vi "commander2.vi"() -> ()   [LabVIEW 2012]
uses:
  G_SEN.vi
  G_LCM.vi
  G_PATH.vi
  G_VEH.vi
  G_NAV.vi
  G_DATA.vi
  <vilib>/Analysis/Matrix/Datatypes/RealMatrix.ctl
  <vilib>/Analysis/Matrix/NI_Matrix.lvlib
panel:
  in  "gain":dbl=0.7
  out "Waveform Chart 8":dbl(graph)
  out "Waveform Chart 7":dbl(graph)
  out "Waveform Chart 6":dbl(graph)
  in  "save lcm":bool
  out "LCM Recv Data":string
  out "GPS DATA 2":T1={"type"="None", "x_lcc"=-59.06772232055664, "y_lcc"=-26.082616806030273, "latdev"=0.0, "londev"=0.0, "sats"=0, "gps_l1_ranges"=0, "gps_l1_mask_ranges"=0, "gps_l2_mask_ranges"=0, "Heading"=89.78975677490234, "lon"=0.0, "lat"=0.0, "time"="None", "hgps"=89.78975677490234, "lag"=89.78975677490234, "MAP"="None"} {"lag" format="%#_5g"; "hgps" format="%#_5g"; "lat" format="%#_11g"; "lon" format="%#_11g"; "Heading" format="%#_5g"; "latdev" format="%#_4g"; "londev" format="%#_4g"}
  in  "obs":bool
  in  "x":dbl
  in  "log":bool
  out "Waveform Chart 5":dbl(graph)
  in  "y":dbl min=-1.0 max=1.0 step=1.0
  out "x = 0?":bool
  out "timmer 2":u32
  out "timmer":u32
  out "Speed limit":dbl=8.0
  out "collision":bool
  out "Mission":i32=9
  in  "Load WPT":bool
  in  "Max. Vel.":dbl=20.0
  in  "RESET PATH":bool
  out "col":i16(graph)
  out "stop":bool
  in  "Reverse":bool
  in  "STOP":bool
  out "Waveform Chart 4":cluster{"auto":i16, "run":i16}(graph)={"auto"=1, "run"=0}
  out "Waveform Chart 3":T2(graph)={"Steer_input"=10.50986504720403, "Steer_output"=3.6, "handle"=10.50986504720403}
  out "Waveform Chart 2":T3(graph)={"VS_des"=4.606086314285715, "VS_can"=8.738, "VS_des"=5.0237113142857135}
  out "Heading":cluster{"Heading":dbl, "hgps":dbl}(graph)={"Heading"=269.76568785604456, "hgps"=270.2149981902155}
  out "XY Graph 2":cluster{"Y":dbl[], "Y":dbl[]}[](graph)=[{"Y"=[-241.57278442382812], "Y"=[-497.6172790527344]}, {"Y"=array[297 elements], "Y"=array[297 elements]}, {"Y"=array[297 elements], "Y"=array[297 elements]}, {"Y"=[-96.81030887093378], "Y"=[-438.1146154201037]}]
  out "Gauge":cluster{dbl, dbl, dbl}(knob)={4.606086314285715, 8.738, 5.0237113142857135} scale=-20.0..140.0
  out "Meter":cluster{dbl, dbl, dbl}(knob)={10.50986504720403, 3.6, 10.50986504720403} scale=-550.0..550.0
  out "XY Graph":cluster{"Y":dbl[], "Y":dbl[]}[](graph)=[{"Y"=[0.0], "Y"=[1000.0]}, {"Y"=[], "Y"=[]}, {"Y"=[], "Y"=[]}, {"Y"=[55.79381017995934], "Y"=[-143.41137512848826]}, {"Y"=[1.8243630881955273], "Y"=[-0.6091599202647308]}, {"Y"=[60.825233010671326, 56.37330625127248, 55.349089235151354, 59.801015994550255, 60.825233010671326], "Y"=[-144.72018116547483, -142.44414335187238, -144.44751039360185, -146.72354820720435, -144.72018116547483]}, {"Y"=[0.0, 2.210107140854234e-06, 8.840428449730098e-06, 1.9890964154001267e-05, 3.536171391260723e-05, 5.5252677611861145e-05, 7.956385525176302e-05, 0.00010829524660493917, 0.00014144685155770276, 0.0001790186695416196, 0.00022101070067037654, 0.00026742294460291305, 0.00031825540077079495, 0.00037350806894664856, 0.0004331809489031002, 0.0004972740399580289, 0.0005657873416566872, 0.0006387208537717015, 0.0007160745756209508, 0.0007978485066360008, 0.0008840426462484174, 0.0009746569938897665, 0.0010696915488779268, 0.0011691463105307776, 0.0012730212781661976, 0.001381316451102066, 0.0014940318285425747, 0.0016111674095782291, 0.0017327231935269083, 0.0018586991794791174, 0.001989095366525362, 0.00212391175364246, 0.002263148340148291, 0.0024068051247922995, 0.002554882106551304, 0.0027073792846294964, 0.002864296657776322, 0.003025634224741225, 0.003191391984614711, 0.0033615699362599116, 0.003536168078198898, 0.0037151864094084885, 0.003898624928524441, 0.004086483634296201, 0.004278762525359525, 0.004475461600350172, 0.0046765808579039, 0.004882120296656467, 0.0050920799150162566, 0.00530645971150534, 0.005525259684645789, 0.005748479832959674, 0.005976120154741693, 0.006208180648513917, 0.006444661312457356, 0.006685562145094082, 0.006930883144491418, 0.007180624309171435, 0.007434785636974084, 0.007693367126535122, 0.007956368775921874, 0.008223790583087975, 0.008495632546100751, 0.008771894663368585, 0.009052576932504053, 0.00933767935191554, 0.009627201919329309, 0.009921144632812684, 0.010219507490205615, 0.010522290489461739, 0.010829493628421005, 0.011141116904923365, 0.011457160316581394, 0.011777623861462416, 0.012102507536951634, 0.012431811341116372, 0.012765535271228146, 0.013103679325240591, 0.0134462435006526, 0.013793227794963059, 0.014144632205784546, 0.014500456730615952, 0.014860701366956164, 0.015225366112190386, 0.015594450963703821, 0.015967955919109045, 0.0163458809754502, 0.016728226130226176, 0.017114991380822175, 0.017506176724168654, 0.0179017821577645, 0.018301807678767545, 0.018706253284335617, 0.019115118971512857, 0.019528404737457095, 0.01994611057932616, 0.02036823649393682, 0.02079478247856059, 0.021225748530014243, 0.02166113464522823, 0.022100940821246695], "Y"=[0.0, 0.05249999993797367, 0.10499999950378934, 0.15749999832528905, 0.2099999960303148, 0.26249999224670867, 0.31499998660231265, 0.3674999787249688, 0.41999996824251923, 0.472499954782806, 0.5249999379736712, 0.577499917442957, 0.6299998928185055, 0.682499863728159, 0.7349998297997596, 0.7874997906611497, 0.8399997459401715, 0.8924996952646672, 0.9449996382624795, 0.9974995745614504, 1.0499995037894228, 1.1024994255742389, 1.1549993395437415, 1.2074992453257731, 1.2599991425481762, 1.3124990308387938, 1.3649989098254687, 1.4174987791360436, 1.4699986383983614, 1.5224984872402658, 1.574998325289599, 1.6274981521742047, 1.6799979675219257, 1.7324977709606055, 1.784997562118088, 1.837497340622216, 1.8899971061008334, 1.9424968581817836, 1.994996596492911, 2.047496320662059, 2.099996030317072, 2.152495725085793, 2.204995404596067, 2.2574950684757384, 2.309994716352652, 2.3624943478546507, 2.414993962609581, 2.467493560245286, 2.519993140389611, 2.5724927026704023, 2.6249922467155042, 2.6774917721527607, 2.7299912786100196, 2.7824907657151243, 2.834990233095921, 2.887489680380256, 2.939989107195975, 2.9924885131709242, 3.0449878979329497, 3.0974872611098974, 3.1499866023296144, 3.2024859212199472, 3.2549852174087435, 3.3074844905238483, 3.3599837401931105, 3.412482966044377, 3.464982167705495, 3.5174813448043127, 3.5699804969686775, 3.6224796238264374, 3.6749787250054404, 3.7274778001335362, 3.7799768488385714, 3.8324758707483966, 3.884974865490859, 3.9374738326938097, 3.989972771985096, 4.042471682992569, 4.094970565344078, 4.147469418667473, 4.199968242590603, 4.2524670367413195, 4.304965800747474, 4.3574645342369145, 4.409963236837495, 4.4624619081770645, 4.514960547883476, 4.567459155584579, 4.6199577309082285, 4.672456273482274, 4.724954782934569, 4.777453258892966, 4.829951700985317, 4.882450108839476, 4.934948482083297, 4.987446820344632, 5.039945123251335, 5.09244339043126, 5.144941621512262, 5.197439816122197, 5.249937973888915]}, {"Y"=[55.85492946607054, 56.300112183962334, 56.74529490185413, 57.19047761974598, 57.635660337637766, 58.08084305552956, 58.52602577342136, 58.97120849131315, 59.416391209205, 59.8615739270968, 60.306756644988596, 60.75193936288038, 61.197122080772175, 61.64230479866403, 62.087487516555825, 62.532670234447615, 62.97785295233941, 63.423035670231265, 63.86821838812306, 64.31340110601485, 64.75858382390665, 65.20376654179844, 65.64894925969023, 66.09413197758208, 66.53931469547388, 66.98449741336567, 67.42968013125746, 67.87486284914931, 68.3200455670411, 68.7652282849329, 69.2104110028247, 69.65559372071655, 70.10077643860835, 70.54595915650015, 70.99114187439193, 71.43632459228371, 71.88150731017556, 72.32669002806736, 72.77187274595916, 73.21705546385095], "Y"=[-143.26925304077835, -143.49687629901547, -143.72449955725253, -143.95212281548962, -144.17974607372668, -144.40736933196374, -144.63499259020085, -144.8626158484379, -145.090239106675, -145.3178623649121, -145.54548562314918, -145.7731088813862, -146.00073213962332, -146.22835539786038, -146.45597865609744, -146.68360191433456, -146.91122517257162, -147.1388484308087, -147.36647168904577, -147.59409494728285, -147.82171820551994, -148.04934146375703, -148.27696472199406, -148.50458798023115, -148.73221123846827, -148.9598344967053, -149.18745775494241, -149.4150810131795, -149.64270427141656, -149.87032752965362, -150.09795078789074, -150.3255740461278, -150.55319730436486, -150.78082056260195, -151.00844382083903, -151.23606707907612, -151.46369033731318, -151.6913135955503, -151.91893685378736, -152.14656011202442]}, {"Y"=[46.95734422441421, 47.0463827596022, 47.13542129479015, 47.224459829978144, 47.31349836516614, 47.40253690035408, 47.49157543554208, 47.58061397073008, 47.669652505918016, 47.75869104110601, 47.84772957629395, 47.936768111481946, 48.02580664666995, 48.11484518185789, 48.20388371704588, 48.292922252233886, 48.381960787421825, 48.47099932260982, 48.56003785779782, 48.64907639298576, 48.73811492817376, 48.827153463361746, 48.91619199854969, 49.00523053373769, 49.09426906892568, 49.18330760411363, 49.272346139301625, 49.361384674489564, 49.45042320967757, 49.53946174486556, 49.6285002800535, 49.717538815241504, 49.8065773504295, 49.89561588561743, 49.984654420805434, 50.07369295599343, 50.16273149118137, 50.251770026369364, 50.34080856155737, 50.429847096745306, 50.5188856319333, 50.607924167121304, 50.69696270230924, 50.78600123749724, 50.875039772685184, 50.96407830787318, 51.05311684306117, 51.142155378249115, 51.23119391343711, 51.320232448625106, 51.40927098381305, 51.49830951900105, 51.58734805418904, 51.67638658937698, 51.765425124564985, 51.85446365975298, 51.94350219494092, 52.03254073012892, 52.12157926531691, 52.21061780050485, 52.29965633569285, 52.38869487088079, 52.477733406068786, 52.56677194125679, 52.65581047644473, 52.74484901163272, 52.833887546820726, 52.922926082008665, 53.01196461719666, 53.10100315238466, 53.190041687572595, 53.27908022276059, 53.36811875794859, 53.45715729313653, 53.54619582832453, 53.635234363512524, 53.72427289870047, 53.813311433888465, 53.902349969076404, 53.99138850426441, 54.0804270394524, 54.16946557464034, 54.25850410982834, 54.34754264501633, 54.43658118020427, 54.525619715392274, 54.61465825058027, 54.70369678576821, 54.792735320956204, 54.88177385614421, 54.970812391332146, 55.05985092652014, 55.148889461708144, 55.23792799689608, 55.32696653208408, 55.41600506727202, 55.50504360246001, 55.59408213764801, 55.683120672835955, 55.77215920802395, 55.861197743211946, 55.95023627839994, 56.03927481358789, 56.12831334877588, 56.21735188396388, 56.306390419151825, 56.39542895433982, 56.48446748952781, 56.573506024715755, 56.66254455990375, 56.75158309509169, 56.84062163027969, 56.92966016546769, 57.01869870065563, 57.10773723584363, 57.196775771031625, 57.285814306219564, 57.37485284140757, 57.46389137659556, 57.552929911783494, 57.64196844697149, 57.73100698215949, 57.82004551734743, 57.90908405253543, 58.08716112291137, 58.176199658099364, 58.26523819328731, 58.354276728475305, 58.4433152636633, 58.53235379885125, 58.62139233403924, 58.71043086922723, 58.79946940441518, 58.88850793960317, 58.97754647479111, 59.06658500997911, 59.15562354516711, 59.24466208035505, 59.333700615543044, 59.42273915073105, 59.511777685918986, 59.60081622110698, 59.689854756294984, 59.778893291482916, 59.86793182667091, 59.956970361858914, 60.04600889704685, 60.13504743223485, 60.31312450261079, 60.402163037798786, 60.491201572986725, 60.58024010817473, 60.66927864336272, 60.75831717855066, 60.84735571373866, 60.93639424892665, 61.02543278411459, 61.114471319302595, 61.203509854490534, 61.29254838967853, 61.38158692486653, 61.47062546005447, 61.55966399524247, 61.64870253043047, 61.73774106561841, 61.826779600806404, 61.91581813599439, 62.00485667118234, 62.093895206370334, 62.18293374155833, 62.271972276746276, 62.36101081193427, 62.45004934712227, 62.53908788231021, 62.62812641749821, 62.71716495268615, 62.80620348787415, 62.895242023062146, 62.984280558250084, 63.07331909343808, 63.162357628626076, 63.251396163814015, 63.34043469900201, 63.42947323419001, 63.51851176937796, 63.60755030456595, 63.69658883975394, 63.78562737494189, 63.87466591012988, 63.96370444531783, 64.05274298050581, 64.14178151569382, 64.23082005088176, 64.31985858606976, 64.40889712125775, 64.4979356564457, 64.58697419163369, 64.76505126200964, 64.85408979719762, 64.94312833238557, 65.03216686757357, 65.12120540276156, 65.2102439379495, 65.29928247313751, 65.38832100832549, 65.47735954351344, 65.56639807870144, 65.65543661388938, 65.74447514907737, 65.83351368426537, 65.92255221945331, 66.0115907546413, 66.10062928982931, 66.18966782501724, 66.27870636020525, 66.36774489539324, 66.45678343058118, 66.54582196576918, 66.63486050095719, 66.72389903614511, 66.81293757133312, 66.9019761065211, 66.99101464170904, 67.08005317689705, 67.16909171208498, 67.25813024727299, 67.34716878246098, 67.43620731764892, 67.52524585283692, 67.61428438802493, 67.70332292321285, 67.79236145840086, 67.88139999358886, 67.97043852877678, 68.05947706396479, 68.14851559915279, 68.23755413434073, 68.32659266952872, 68.41563120471668, 68.50466973990466, 68.59370827509267, 68.6827468102806, 68.7717853454686, 68.8608238806566, 68.94986241584455, 69.03890095103253, 69.12793948622053, 69.21697802140848, 69.30601655659646, 69.39505509178447, 69.48409362697241, 69.5731321621604, 69.6621706973484, 69.75120923253635, 69.84024776772434, 69.92928630291229, 70.01832483810027, 70.10736337328828, 70.19640190847622, 70.2854404436642, 70.37447897885221, 70.46351751404015, 70.55255604922814, 70.64159458441614, 70.7306331196041, 70.81967165479207, 70.90871018998008, 70.99774872516802, 71.08678726035602, 71.17582579554401, 71.26486433073195, 71.35390286591995, 71.44294140110789, 71.5319799362959, 71.62101847148388, 71.71005700667183, 71.79909554185983, 71.88813407704782, 71.97717261223576, 72.06621114742377, 72.15524968261175, 72.2442882177997, 72.3333267529877, 72.42236528817568, 72.51140382336364, 72.60044235855163, 72.68948089373963, 72.77851942892757, 72.86755796411556, 72.9565964993035, 73.04563503449151, 73.13467356967949, 73.22371210486745, 73.31275064005544, 73.40178917524342, 73.49082771043138, 73.57986624561937], "Y"=[-138.89375124553214, -138.93927200180423, -138.98479275807625, -139.0303135143483, -139.07583427062036, -139.12135502689242, -139.16687578316444, -139.21239653943653, -139.25791729570855, -139.30343805198058, -139.34895880825266, -139.3944795645247, -139.44000032079677, -139.4855210770688, -139.53104183334085, -139.5765625896129, -139.62208334588496, -139.667604102157, -139.71312485842907, -139.7586456147011, -139.80416637097318, -139.8496871272452, -139.89520788351723, -139.9407286397893, -139.98624939606134, -140.0317701523334, -140.07729090860545, -140.1228116648775, -140.16833242114956, -140.2138531774216, -140.25937393369364, -140.30489468996572, -140.35041544623775, -140.39593620250977, -140.44145695878186, -140.48697771505388, -140.53249847132597, -140.578019227598, -140.62353998387005, -140.66906074014207, -140.71458149641416, -140.76010225268618, -140.80562300895826, -140.8511437652303, -140.89666452150234, -140.9421852777744, -140.98770603404643, -141.0332267903185, -141.07874754659053, -141.1242683028626, -141.16978905913462, -141.2153098154067, -141.26083057167872, -141.3063513279508, -141.35187208422283, -141.3973928404949, -141.44291359676694, -141.48843435303897, -141.53395510931105, -141.57947586558308, -141.62499662185516, -141.67051737812716, -141.71603813439924, -141.76155889067127, -141.80707964694335, -141.85260040321535, -141.89812115948743, -141.94364191575949, -141.9891626720315, -142.0346834283036, -142.08020418457562, -142.1257249408477, -142.1712456971197, -142.21676645339178, -142.2622872096638, -142.3078079659359, -142.3533287222079, -142.39884947847997, -142.44437023475203, -142.48989099102408, -142.53541174729614, -142.58093250356816, -142.62645325984025, -142.67197401611224, -142.71749477238433, -142.76301552865635, -142.80853628492844, -142.85405704120046, -142.89957779747255, -142.94509855374454, -142.99061931001663, -143.03614006628868, -143.0816608225607, -143.1271815788328, -143.17270233510482, -143.2182230913769, -143.2637438476489, -143.30926460392098, -143.354785360193, -143.4003061164651, -143.4458268727371, -143.4913476290092, -143.5368683852812, -143.58238914155328, -143.62790989782533, -143.67343065409736, -143.71895141036944, -143.76447216664147, -143.80999292291352, -143.85551367918555, -143.90103443545763, -143.94655519172966, -143.99207594800174, -144.03759670427374, -144.08311746054582, -144.12863821681785, -144.1741589730899, -144.21967972936199, -144.265200485634, -144.3107212419061, -144.3562419981781, -144.40176275445017, -144.4472835107222, -144.49280426699428, -144.58384577953836, -144.6293665358104, -144.67488729208247, -144.72040804835453, -144.76592880462653, -144.81144956089864, -144.85697031717064, -144.90249107344272, -144.94801182971474, -144.99353258598683, -145.03905334225882, -145.0845740985309, -145.13009485480293, -145.17561561107502, -145.22113636734704, -145.2666571236191, -145.31217787989118, -145.35769863616318, -145.40321939243526, -145.4487401487073, -145.49426090497937, -145.5397816612514, -145.58530241752348, -145.63082317379548, -145.7218646863396, -145.76738544261164, -145.8129061988837, -145.85842695515572, -145.90394771142783, -145.94946846769983, -145.9949892239719, -146.04050998024394, -146.08603073651602, -146.13155149278802, -146.1770722490601, -146.22259300533213, -146.2681137616042, -146.31363451787624, -146.3591552741483, -146.40467603042035, -146.45019678669237, -146.49571754296446, -146.54123829923648, -146.58675905550857, -146.6322798117806, -146.67780056805265, -146.72332132432467, -146.76884208059676, -146.81436283686878, -146.85988359314084, -146.9054043494129, -146.95092510568492, -146.99644586195703, -147.04196661822903, -147.0874873745011, -147.13300813077313, -147.17852888704522, -147.22404964331722, -147.2695703995893, -147.31509115586132, -147.3606119121334, -147.40613266840543, -147.4516534246775, -147.49717418094954, -147.54269493722157, -147.58821569349365, -147.63373644976568, -147.67925720603776, -147.72477796230976, -147.77029871858184, -147.81581947485387, -147.86134023112595, -147.90686098739798, -147.9979024999421, -148.0434232562141, -148.08894401248617, -148.13446476875822, -148.17998552503028, -148.22550628130233, -148.27102703757438, -148.3165477938464, -148.3620685501185, -148.40758930639052, -148.45311006266255, -148.49863081893463, -148.54415157520666, -148.58967233147874, -148.63519308775076, -148.6807138440228, -148.72623460029487, -148.77175535656693, -148.81727611283895, -148.86279686911104, -148.90831762538306, -148.95383838165512, -148.99935913792717, -149.0448798941992, -149.09040065047128, -149.1359214067433, -149.18144216301536, -149.22696291928742, -149.27248367555944, -149.31800443183153, -149.36352518810358, -149.4090459443756, -149.4545667006477, -149.50008745691972, -149.54560821319174, -149.59112896946382, -149.63664972573585, -149.68217048200793, -149.72769123827996, -149.77321199455199, -149.81873275082407, -149.86425350709612, -149.90977426336815, -149.95529501964023, -150.00081577591226, -150.0463365321843, -150.09185728845637, -150.1373780447284, -150.18289880100048, -150.2284195572725, -150.27394031354456, -150.3194610698166, -150.36498182608864, -150.4105025823607, -150.45602333863278, -150.5015440949048, -150.54706485117688, -150.5925856074489, -150.63810636372094, -150.68362711999302, -150.72914787626505, -150.7746686325371, -150.82018938880915, -150.86571014508118, -150.91123090135326, -150.9567516576253, -151.00227241389734, -151.04779317016943, -151.09331392644145, -151.13883468271348, -151.18435543898556, -151.2298761952576, -151.27539695152967, -151.3209177078017, -151.36643846407375, -151.4119592203458, -151.45747997661783, -151.5030007328899, -151.54852148916194, -151.594042245434, -151.63956300170608, -151.6850837579781, -151.73060451425013, -151.77612527052221, -151.82164602679424, -151.8671667830663, -151.91268753933835, -151.95820829561038, -152.00372905188246, -152.04924980815449, -152.09477056442654, -152.14029132069862, -152.18581207697065, -152.23133283324267, -152.27685358951476, -152.32237434578678, -152.36789510205887, -152.4134158583309, -152.45893661460295, -152.504457370875]}, {"Y"=[], "Y"=[]}, {"Y"=[], "Y"=[]}, {"Y"=[], "Y"=[]}, {"Y"=[-16.5, -15.25, -15.0, -13.5, -13.25, -13.25, -13.25, -13.0, -13.0, -12.75, -12.75, -12.75, -12.75, -12.75, -12.75, -12.75, -12.5, -12.5, -12.5, -12.5, -12.5, -12.5, -12.25, -12.25, -12.25, -12.25, -12.25, -12.25, -12.0, -12.0, -12.0, -11.75, -11.75, -11.75, -11.5, -11.5, -11.5, -11.5, -11.5, -11.25, -10.75, -10.75, -10.5, -10.5, -10.25, -10.25, -10.0, -10.0, -10.0, -10.0, -10.0, -9.75, -9.75, -9.75, -9.75, -9.75, -9.75, -9.75, -9.75, -9.75, -9.75, -9.5, -9.5, -9.5, -9.5, -9.5, -9.5, -9.5, -9.5, -9.5, -9.5, -9.5, -9.5, -9.5, -9.5, -9.5, -9.5, -9.5, -9.5, -9.5, -9.25, -9.25, -9.25, -9.25, -9.25, -9.25, -9.25, -9.25, -9.25, -9.25, -9.25, -9.25, -9.25, -9.25, -9.25, -9.25, -9.25, -9.25, -9.25, -9.25, -9.25, -9.25, -9.0, -9.0, -9.0, -9.0, -9.0, -9.0, -9.0, -9.0, -9.0, -9.0, -9.0, -9.0, -9.0, -9.0, -9.0, -9.0, -9.0, -9.0, -9.0, -9.0, -9.0, -9.0, -9.0, -9.0, -9.0, -9.0, -8.75, -8.75, -8.75, -8.75, -8.75, -8.75, -8.75, -8.75, -8.75, -8.75, -8.75, -8.75, -8.75, -8.75, -8.75, -8.75, -8.75, -8.75, -8.75, -8.75, -8.75, -8.75, -8.75, -8.75, -8.75, -8.75, -8.75, -8.75, -8.75, -8.75, -8.75, -8.75, -8.75, -8.75, -8.75, -8.75, -8.75, -8.5, -8.5, -8.5, -8.5, -8.5, -8.5, -8.5, -8.5, -8.5, -8.5, -8.5, -8.5, -8.5, -8.5, -8.5, -8.5, -8.5, -8.5, -8.5, -8.5, -8.5, -8.5, -8.5, -8.5, -8.5, -8.5, -8.5, -8.5, -8.5, -8.5, -8.5, -8.5, -8.5, -8.5, -8.5, -8.5, -8.25, -8.25, -8.25, -8.25, -8.25, -8.25, -8.25, -8.25, -8.25, -8.25, -8.25, -8.25, -8.25, -8.25, -8.25, -8.25, -8.25, -8.25, -8.25, -8.25, -8.25, -8.25, -8.25, -8.25, -8.25, -8.25, -8.25, -8.25, -8.25, -8.25, -8.25, -8.25, -8.25, -8.0, -8.0, -8.0, -8.0, -8.0, -8.0, -8.0, -8.0, -8.0, -8.0, -8.0, -8.0, -8.0, -8.0, -8.0, -8.0, -8.0, -8.0, -8.0, -8.0, -8.0, -8.0, -8.0, -8.0, -8.0, -7.75, -7.75, -7.75, -7.75, -7.75, -7.75, -7.75, -7.75, -7.75, -7.75, -7.75, -7.75, -7.75, -7.75, -7.75, -7.75, -7.75, -7.75, -7.75, -7.75, -7.75, -7.75, -7.75, -7.75, -7.75, -7.75, -7.5, -7.5, -7.5, -7.5, -7.5, -7.5, -7.5, -7.5, -7.5, -7.5, -7.5, -7.5, -7.5, -7.5, -7.5, -7.5, -7.5, -7.5, -7.5, -7.5, -7.5, -7.5, -7.5, -7.5, -7.5, -7.25, -7.25, -7.25, -7.25, -7.25, -7.25, -7.25, -7.25, -7.25, -7.25, -7.25, -7.25, -7.25, -7.25, -7.25, -7.25, -7.25, -7.25, -7.25, -7.25, -7.25, -7.25, -7.25, -7.0, -7.0, -7.0, -7.0, -7.0, -7.0, -7.0, -7.0, -7.0, -7.0, -7.0, -7.0, -7.0, -7.0, -7.0, -7.0, -7.0, -7.0, -7.0, -6.75, -6.75, -6.75, -6.75, -6.75, -6.75, -6.75, -6.75, -6.75, -6.75, -6.75, -6.75, -6.75, -6.75, -6.75, -6.75, -6.75, -6.75, -6.75, -6.75, -6.75, -6.75, -6.75, -6.5, -6.5, -6.5, -6.5, -6.5, -6.5, -6.5, -6.5, -6.5, -6.5, -6.5, -6.5, -6.5, -6.5, -6.5, -6.5, -6.5, -6.5, -6.5, -6.5, -6.5, -6.5, -6.5, -6.5, -6.5, -6.5, -6.5, -6.5, -6.5, -6.5, -6.25, -6.25, -6.25, -6.25, -6.25, -6.25, -6.25, -6.25, -6.25, -6.25, -6.25, -6.25, -6.25, -6.25, -6.25, -6.25, -6.25, -6.0, -6.0, -6.0, -6.0, -6.0, -6.0, -6.0, -6.0, -6.0, -6.0, -6.0, -5.75, -5.75, -5.75, -5.75, -5.75, -5.75, -5.75, -5.75, -5.75, -5.75, -5.5, -5.25, -5.0, -4.75, -4.5, -4.5, -4.25, -4.25, -4.0, -4.0, -3.75, -3.75, -3.5, -3.5, -3.25, -3.25, -3.25, -3.25, -3.0, -3.0, 2.0, 2.0, 2.0, 2.0, 2.0, 2.0, 2.0, 2.25, 2.25, 2.25, 2.25, 2.25, 2.25, 2.25, 2.25, 2.25, 2.25, 2.25, 2.25, 2.25, 2.25, 2.25, 2.25, 2.25, 2.25, 2.25, 2.25, 2.25, 2.25, 2.5, 2.5, 2.5, 2.5, 2.5, 2.5, 2.5, 2.5, 2.5, 2.5, 2.5, 2.5, 2.5, 2.5, 2.5, 2.5, 2.5, 2.5, 2.5, 2.5, 2.5, 2.5, 2.5, 2.5, 2.5, 2.5, 2.5, 2.5, 2.5, 2.5, 2.5, 2.5, 2.5, 2.5, 2.5, 2.5, 2.5, 2.5, 2.5, 2.5, 2.5, 2.5, 2.75, 2.75, 2.75, 2.75, 2.75, 2.75, 2.75, 2.75, 2.75, 2.75, 2.75, 2.75, 2.75, 2.75, 2.75, 2.75, 2.75, 2.75, 2.75, 2.75, 2.75, 2.75, 2.75, 2.75, 2.75, 2.75, 2.75, 2.75, 2.75, 2.75, 2.75, 2.75, 2.75, 2.75, 2.75, 2.75, 2.75, 2.75, 2.75, 2.75, 2.75, 2.75, 2.75, 2.75, 2.75, 2.75, 2.75, 2.75, 2.75, 2.75, 3.0, 3.0, 3.0, 3.0, 3.0, 3.0, 3.0, 3.0, 3.0, 3.0, 3.0, 3.0, 3.0, 3.0, 3.0, 3.0, 3.0, 3.0, 3.0, 3.0, 3.0, 3.0, 3.0, 3.0, 3.0, 3.0, 3.0, 3.0, 3.0, 3.0, 3.0, 3.0, 3.0, 3.0, 3.0, 3.0, 3.0, 3.0, 3.0, 3.0, 3.0, 3.0, 3.0, 3.0, 3.0, 3.0, 3.0, 3.25, 3.25, 3.25, 3.25, 3.25, 3.25, 3.25, 3.25, 3.25, 3.25, 3.25, 3.25, 3.25, 3.25, 3.25, 3.25, 3.25, 3.25, 3.25, 3.25, 3.25, 3.25, 3.25, 3.25, 3.25, 3.25, 3.25, 3.25, 3.25, 3.25, 3.25, 3.25, 3.25, 3.25, 3.25, 3.25, 3.25, 3.25, 3.25, 3.25, 3.25, 3.25, 3.25, 3.25, 3.25, 3.25, 3.25, 3.25, 3.25, 3.25, 3.25, 3.25, 3.25, 3.5, 3.5, 3.5, 3.5, 3.5, 3.5, 3.5, 3.5, 3.5, 3.5, 3.5, 3.5, 3.5, 3.5, 3.5, 3.5, 3.5, 3.5, 3.5, 3.5, 3.5, 3.5, 3.5, 3.5, 3.5, 3.5, 3.5, 3.5, 3.5, 3.5, 3.5, 3.5, 3.5, 3.5, 3.5, 3.5, 3.5, 3.5, 3.5, 3.5, 3.5, 3.5, 3.5, 3.5, 3.5, 3.5, 3.5, 3.5, 3.5, 3.5, 3.5, 3.5, 3.5, 3.5, 3.5, 3.5, 3.5, 3.75, 3.75, 3.75, 3.75, 3.75, 3.75, 3.75, 3.75, 3.75, 3.75, 3.75, 3.75, 3.75, 3.75, 3.75, 3.75, 3.75, 3.75, 3.75, 3.75, 3.75, 3.75, 3.75, 3.75, 3.75, 3.75, 3.75, 3.75, 3.75, 3.75, 3.75, 3.75, 3.75, 3.75, 3.75, 3.75, 3.75, 4.0, 4.0, 4.0, 4.0, 4.0, 4.0, 4.0, 4.0, 4.0, 4.0, 4.0, 4.0, 4.0, 4.0, 4.0, 4.0, 4.0, 4.0, 4.0, 4.0, 4.0, 4.0, 4.0, 4.0, 4.0, 4.0, 4.0, 4.0, 4.0, 4.0, 4.0, 4.0, 4.0, 4.0, 4.0, 4.0, 4.25, 4.25, 4.25, 4.25, 4.25, 4.25, 4.25, 4.25, 4.25, 4.25, 4.25, 4.25, 4.25, 4.25, 4.25, 4.25, 4.25, 4.25, 4.25, 4.25, 4.25, 4.25, 4.25, 4.25, 4.25, 4.25, 4.25, 4.25, 4.25, 4.25, 4.25, 4.25, 4.25, 4.25, 4.25, 4.25, 4.25, 4.25, 4.25, 4.25, 4.25, 4.25, 4.25, 4.5, 4.5, 4.5, 4.5, 4.5, 4.5, 4.5, 4.5, 4.5, 4.5, 4.5, 4.5, 4.5, 4.5, 4.5, 4.5, 4.5, 4.5, 4.5, 4.5, 4.5, 4.5, 4.5, 4.5, 4.5, 4.5, 4.5, 4.75, 4.75, 4.75, 4.75, 4.75, 4.75, 4.75, 4.75, 4.75, 4.75, 4.75, 4.75, 4.75, 4.75, 4.75, 4.75, 4.75, 4.75, 4.75, 4.75, 4.75, 4.75, 4.75, 4.75, 4.75, 4.75, 4.75, 4.75, 4.75, 5.0, 5.0, 5.0, 5.0, 5.0, 5.0, 5.0, 5.0, 5.0, 5.0, 5.0, 5.0, 5.0, 5.0, 5.0, 5.0, 5.0, 5.0, 5.0, 5.0, 5.0, 5.25, 5.25, 5.25, 5.25, 5.25, 5.25, 5.25, 5.25, 5.25, 5.25, 5.25, 5.25, 5.25, 5.25, 5.5, 5.5, 5.5, 5.5, 5.5, 5.5, 5.5, 5.5, 5.5, 5.5, 5.5, 5.5, 5.75, 5.75, 5.75, 5.75, 5.75, 5.75, 5.75, 5.75, 5.75, 5.75, 5.75, 5.75, 5.75, 5.75, 5.75, 5.75, 5.75, 6.0, 6.0, 6.0, 6.0, 6.0, 6.0, 6.0, 6.0, 6.0, 6.0, 6.0, 6.25, 6.25, 6.25, 6.25, 6.25, 6.25, 6.25, 6.25, 6.5, 6.5, 6.5, 6.5, 6.5, 6.5, 6.5, 6.5, 6.5, 6.75, 6.75, 6.75, 6.75, 7.0, 7.0, 7.0, 7.25, 7.25, 7.25, 7.25, 7.25, 7.25, 7.25, 7.5, 7.5, 8.0, 8.0, 8.0, 8.0, 8.0, 8.25, 8.25, 8.5, 8.5, 8.5, 8.75, 8.75, 8.75, 8.75, 8.75, 9.0, 9.0, 9.0, 9.0, 9.0, 9.0, 9.25, 9.25, 9.25, 9.25, 9.25, 9.25, 9.5, 9.5, 9.5, 9.5, 9.5, 9.5, 9.75, 9.75, 9.75, 10.0, 10.0, 10.0, 10.0, 10.25, 10.25, 10.5, 10.5, 10.5, 10.75, 10.75, 10.75, 10.75, 11.0, 11.0, 11.0, 11.0, 11.0, 11.25, 11.25, 11.25, 11.25, 11.25, 11.25, 11.25, 11.25, 11.25, 11.25, 11.5, 11.5, 11.5, 11.5, 11.5, 11.5, 11.5, 11.5, 11.5, 11.5, 11.5, 11.5, 11.5, 11.5, 11.5, 11.75, 11.75, 11.75, 11.75, 11.75, 11.75, 11.75, 11.75, 11.75, 11.75, 11.75, 11.75, 11.75, 11.75, 11.75, 11.75, 11.75, 11.75, 11.75, 11.75, 12.0, 12.0, 12.0, 12.0, 12.0, 12.0, 12.0, 12.0, 12.0, 12.0, 12.0, 12.0, 12.0, 12.0, 12.0, 12.0, 12.0, 12.0, 12.0, 12.0, 12.0, 12.0, 12.0, 12.0, 12.0, 12.0, 12.0, 12.25, 12.25, 12.25, 12.25, 12.25, 12.25, 12.25, 12.25, 12.25, 12.25, 12.25, 12.25, 12.25, 12.25, 12.25, 12.25, 12.5, 12.5, 12.5, 12.5, 12.5, 12.5, 12.5, 12.5, 12.5, 12.5, 12.5, 12.5, 12.5, 12.75, 12.75, 12.75, 12.75, 12.75, 12.75, 12.75, 12.75, 12.75, 12.75, 13.0, 13.0, 13.0, 13.0, 13.0, 13.0, 13.0, 13.0, 13.0, 13.0, 13.0, 13.0, 13.0, 13.0, 13.0, 13.0, 13.0, 13.0, 13.0, 13.0, 13.0, 13.0, 13.0, 13.25, 13.25, 13.25, 13.25, 13.25, 13.25, 13.25, 13.25, 13.25, 13.25, 13.25, 13.25, 13.25, 13.25, 13.25, 13.25, 13.25, 13.25, 13.25, 13.5, 13.5, 13.5, 13.5, 13.5, 13.5, 13.5, 13.5, 13.5, 13.5, 13.75, 13.75, 13.75, 13.75, 13.75, 13.75, 13.75, 13.75, 13.75, 14.0, 14.0, 14.0, 14.0, 14.5, 14.75, 15.5, 15.75, 16.0, 19.25, 19.25, 19.25, 19.5, 19.5, 19.75, 22.25, 22.25, 22.25, 22.5, 22.5, 22.5, 22.75, 22.75, 22.75, 22.75, 23.0, 23.0, 23.0, 23.25, 23.25, 23.25, 23.5, 23.5, 23.5, 23.5, 23.5, 23.5, 23.75, 23.75, 23.75, 23.75, 23.75, 23.75, 23.75, 23.75, 23.75, 23.75, 23.75, 24.0, 24.0, 24.0, 24.0, 24.0, 24.0, 24.0, 24.25, 24.25, 24.5], "Y"=[46.5, 46.5, 46.5, 2.75, 0.5, 2.75, 17.0, 0.75, 17.25, -6.5, -2.25, -1.75, 0.5, 0.75, 1.0, 3.75, -6.5, 0.75, 4.0, 4.25, 17.25, 21.5, -6.75, -6.5, -1.75, 17.25, 21.5, 22.25, -6.75, 21.75, 22.0, -6.5, 11.25, 22.0, 10.5, 10.75, 11.0, 11.5, 11.75, -6.0, 3.75, 8.25, -1.0, 8.25, -1.25, -1.0, -7.0, -1.25, 2.75, 3.0, 3.5, -10.75, -10.5, -10.0, -9.5, -9.25, -8.25, -6.75, -1.25, 3.0, 3.25, -20.5, -15.5, -15.25, -14.75, -10.5, -10.25, -10.0, -9.75, -9.25, -9.0, -8.75, -8.25, -8.0, -7.75, -7.5, -1.0, 0.5, 1.5, 2.75, -20.25, -18.25, -17.75, -17.5, -17.0, -15.75, -15.5, -10.75, -10.25, -9.5, -9.0, -8.75, -8.25, -8.0, -7.75, 0.75, 1.0, 1.25, 2.25, 3.5, 7.25, 7.5, -19.0, -17.5, -17.25, -10.5, -10.25, -10.0, -9.25, -9.0, -8.75, -8.25, -8.0, -7.25, -7.0, -6.75, -4.75, -4.5, -4.25, 0.75, 1.0, 1.25, 1.75, 2.25, 2.5, 2.75, 3.5, 7.5, -17.5, -12.75, -12.0, -11.75, -10.5, -9.75, -9.5, -9.25, -9.0, -8.75, -8.5, -8.25, -8.0, -7.75, -7.5, -7.0, -6.75, -4.75, -4.5, -3.75, -3.25, -3.0, -1.5, -0.5, -0.25, 0.0, 0.25, 1.75, 2.5, 2.75, 4.25, 4.75, 5.5, 5.75, 6.25, 7.5, 7.75, -13.25, -13.0, -12.75, -12.0, -11.75, -8.25, -8.0, -7.0, -6.75, -5.5, -5.0, -4.75, -4.5, -4.0, -3.75, -3.25, -3.0, -2.75, -2.0, -1.75, -1.5, -1.0, -0.5, -0.25, 0.0, 0.25, 0.5, 0.75, 1.75, 2.0, 4.0, 4.25, 4.75, 5.75, 6.0, 6.25, -17.5, -12.75, -12.0, -11.5, -10.25, -8.25, -8.0, -7.75, -5.5, -4.75, -4.0, -3.75, -3.5, -3.25, -3.0, -2.75, -2.5, -2.25, -2.0, -1.75, -1.5, -0.75, -0.5, -0.25, 0.0, 0.25, 0.5, 2.25, 4.5, 4.75, 5.75, 6.0, 6.25, -13.5, -13.25, -13.0, -7.75, -5.75, -5.5, -5.25, -5.0, -4.75, -4.5, -3.75, -3.5, -3.25, -2.25, -2.0, -1.75, -1.5, -1.25, -0.75, -0.5, -0.25, 0.0, 0.25, 0.5, 0.75, -13.25, -12.5, -6.0, -5.75, -5.25, -5.0, -4.75, -4.5, -4.25, -3.25, -2.5, -2.25, -2.0, -1.75, -1.5, -1.25, -0.75, -0.5, -0.25, 0.0, 0.25, 0.5, 4.0, 4.25, 7.75, 8.0, -14.0, -13.25, -13.0, -8.0, -5.25, -5.0, -4.75, -3.75, -3.0, -2.0, -1.75, -1.5, -1.25, -0.5, -0.25, 0.25, 0.5, 0.75, 1.0, 1.25, 1.5, 2.25, 2.5, 3.75, 9.25, -7.75, -7.25, -7.0, -6.75, -6.5, -6.25, -6.0, -5.75, -5.5, -5.25, -5.0, -3.5, -1.75, -1.5, -1.25, -0.5, -0.25, 1.0, 1.25, 1.75, 2.5, 5.75, 8.5, -9.0, -8.0, -7.75, -7.0, -6.75, -6.5, -5.5, -5.25, -5.0, -2.0, -1.75, 1.25, 1.5, 2.5, 4.0, 4.25, 4.5, 6.0, 8.5, -9.25, -9.0, -7.5, -7.25, -5.75, -5.5, -2.75, -2.5, -1.0, -0.75, -0.5, -0.25, 0.0, 1.0, 1.25, 1.75, 2.75, 3.0, 4.5, 4.75, 5.75, 6.0, 6.25, -20.0, -8.0, -7.5, -7.25, -4.5, -4.25, -3.25, -3.0, -2.75, -2.5, -1.25, -1.0, -0.75, -0.5, 2.25, 2.5, 2.75, 3.0, 3.25, 3.5, 3.75, 4.0, 4.25, 4.5, 4.75, 5.0, 5.25, 5.5, 5.75, 6.0, -20.25, -20.0, -14.0, -13.75, -8.0, -7.75, -7.25, -5.0, -4.75, -4.5, -3.5, -3.25, -3.0, -2.0, -1.75, -1.5, 3.0, -20.0, -14.0, -13.75, -8.0, -7.75, -7.5, -7.25, -5.0, -2.0, -1.75, -1.5, -20.5, -20.25, -14.25, -8.0, -7.75, -7.5, -2.0, -1.75, -1.5, 3.0, 3.0, 3.0, 3.0, 3.0, 3.0, 20.75, 3.0, 20.75, 3.0, 20.75, 3.0, 20.75, 3.0, 20.75, 3.0, 21.0, 22.0, 22.25, 3.0, 22.25, -8.25, -8.0, -7.25, -2.75, -2.5, -2.25, -2.0, -20.5, -14.5, -14.25, -8.5, -8.25, -8.0, -7.75, -7.25, -4.5, -4.0, -3.5, -3.25, -3.0, -2.5, -2.25, -2.0, -1.5, -1.25, -1.0, 4.75, 6.0, 6.25, -20.5, -20.25, -14.25, -8.25, -8.0, -7.75, -5.0, -4.5, -4.25, -4.0, -3.75, -3.5, -3.25, -3.0, -2.75, -2.5, -2.25, -2.0, -1.75, -1.5, -1.25, -1.0, -0.75, 0.75, 1.75, 2.0, 2.25, 2.5, 2.75, 3.0, 3.25, 3.5, 3.75, 4.0, 5.0, 5.25, 5.5, 5.75, 6.25, 6.5, 6.75, 7.0, -20.5, -20.25, -14.25, -8.25, -7.75, -4.75, -4.5, -4.25, -4.0, -3.75, -3.5, -3.25, -3.0, -2.75, -2.5, -2.0, -1.75, -1.5, -1.25, -1.0, -0.75, -0.5, 0.25, 0.5, 0.75, 1.0, 1.25, 1.5, 1.75, 2.0, 2.25, 2.5, 2.75, 3.25, 3.5, 3.75, 4.0, 4.25, 4.5, 4.75, 5.0, 5.25, 5.5, 5.75, 6.0, 6.25, 6.5, 6.75, 7.0, 7.25, -20.25, -7.75, -5.25, -4.5, -4.25, -4.0, -3.75, -3.5, -3.25, -2.75, -2.5, -2.25, -2.0, -1.75, -1.5, -1.25, -1.0, -0.75, -0.5, -0.25, 0.0, 0.25, 0.5, 0.75, 1.0, 1.25, 1.5, 1.75, 2.0, 2.25, 2.5, 2.75, 4.25, 4.5, 4.75, 5.0, 5.25, 5.5, 5.75, 6.0, 6.25, 6.5, 6.75, 7.0, 7.5, 9.5, 10.75, -20.5, -7.5, -6.75, -6.0, -5.75, -5.0, -4.75, -4.5, -4.25, -4.0, -3.25, -3.0, -2.75, -2.5, -2.0, -1.75, -1.5, -1.25, -1.0, -0.75, -0.5, -0.25, 0.0, 0.25, 0.5, 0.75, 1.0, 1.25, 1.5, 1.75, 2.0, 2.25, 2.5, 2.75, 3.0, 4.5, 4.75, 5.0, 5.25, 5.5, 5.75, 6.0, 6.25, 6.5, 6.75, 7.0, 7.25, 9.25, 9.5, 10.75, 11.0, 12.25, 12.75, -7.75, -7.5, -6.75, -6.5, -5.75, -5.5, -5.25, -4.75, -4.25, -4.0, -3.5, -3.0, -2.75, -2.25, -2.0, -1.75, -1.5, -1.25, -1.0, -0.75, -0.5, -0.25, 0.0, 0.25, 0.5, 0.75, 1.0, 1.25, 1.5, 1.75, 2.0, 2.25, 2.5, 2.75, 3.0, 4.75, 5.0, 5.25, 5.5, 5.75, 6.0, 6.5, 6.75, 7.0, 8.75, 9.0, 9.25, 10.25, 10.75, 11.0, 11.25, 12.25, 12.5, 12.75, 13.0, 13.25, 13.75, -8.75, -7.5, -6.5, -6.25, -5.5, -5.0, -4.75, -4.5, -4.25, -4.0, -2.25, -1.75, -1.5, -1.25, -1.0, -0.75, -0.5, -0.25, 0.0, 0.25, 0.5, 1.0, 1.25, 1.5, 1.75, 2.0, 2.25, 2.5, 2.75, 3.0, 3.25, 9.75, 11.0, 11.25, 12.25, 12.5, 13.0, -8.5, -7.5, -6.75, -6.5, -5.5, -5.25, -4.25, -4.0, -3.25, -3.0, -2.75, -2.5, -2.25, -1.75, -1.5, -1.25, -1.0, -0.75, -0.5, -0.25, 0.0, 0.25, 0.5, 0.75, 1.0, 1.25, 1.5, 1.75, 2.0, 2.25, 2.5, 2.75, 3.0, 12.5, 13.0, 13.25, -9.75, -9.5, -9.25, -8.75, -8.5, -8.25, -7.75, -7.5, -7.25, -7.0, -6.75, -6.5, -6.25, -6.0, -5.75, -5.0, -4.25, -3.0, -2.75, -2.5, -2.25, -1.75, -1.5, 0.0, 0.25, 0.5, 0.75, 1.0, 1.25, 1.5, 1.75, 2.0, 2.5, 2.75, 3.0, 3.25, 11.0, 11.25, 11.5, 12.0, 12.25, 12.5, 13.0, -10.0, -9.0, -8.75, -8.5, -8.25, -7.5, -7.25, -6.5, -6.0, -5.75, -4.5, -4.25, -4.0, -3.0, 0.25, 0.5, 0.75, 1.0, 2.5, 2.75, 3.0, 3.5, 11.5, 11.75, 12.0, 12.25, 12.75, -11.25, -10.75, -10.0, -9.5, -9.25, -9.0, -8.75, -8.0, -7.25, -7.0, -6.5, -6.25, -6.0, -5.75, -5.5, -4.75, -4.5, -4.25, -4.0, -3.75, 2.25, 2.5, 2.75, 3.0, 3.5, 6.75, 11.25, 11.5, 12.0, -12.25, -9.0, -8.75, -6.5, -6.25, -6.0, -5.75, -5.5, -5.25, -5.0, -4.75, -4.25, -4.0, -3.75, -3.5, 1.25, 2.5, 2.75, 3.25, 6.75, 12.0, -9.0, -8.75, -8.5, -7.0, -5.75, -5.5, -4.25, -3.5, -3.25, -3.0, -0.75, 2.0, 2.25, 12.0, -10.75, -9.0, -8.25, -3.25, -3.0, 2.0, 2.25, 2.5, 4.25, 5.75, 12.0, 13.0, -9.0, -3.5, 1.0, 1.25, 1.5, 1.75, 2.25, 2.5, 2.75, 3.25, 5.5, 5.75, 8.25, 8.5, 8.75, 9.0, 9.25, -9.0, -8.75, 1.5, 1.75, 3.25, 3.5, 5.5, 5.75, 6.25, 8.25, 9.0, -9.0, -8.75, 1.75, 3.25, 3.75, 5.75, 9.0, 9.5, -17.25, 1.5, 1.75, 3.25, 4.75, 5.5, 6.0, 6.25, 6.75, 4.5, 4.75, 5.5, 6.25, 4.5, 4.75, 5.75, 4.5, 6.25, 8.75, 9.0, 10.25, 10.5, 17.0, 4.0, 17.0, 1.5, 6.75, 10.75, 11.0, 17.5, 0.0, 17.5, 3.25, 17.25, 17.5, 0.25, 3.0, 3.25, 11.25, 11.5, -0.5, 6.75, 11.25, 11.5, 12.25, 35.5, -11.25, 12.0, 12.25, 12.75, 17.0, 35.5, -13.0, -12.25, -10.75, 12.0, 12.25, 17.0, 16.5, 16.75, 28.5, 16.25, 16.5, 28.25, 28.75, 28.0, 28.5, 2.25, 28.0, 28.25, 2.0, 2.5, 3.25, 8.0, 2.75, 3.25, 8.0, 8.25, 15.75, -7.75, -7.5, -5.25, -4.75, -2.25, 5.25, 8.0, 8.25, 15.25, 15.5, -9.25, -7.25, -4.75, -3.5, -3.0, -2.5, 2.5, 4.0, 4.25, 4.5, 4.75, 7.0, 7.75, 8.75, 9.0, -7.75, 1.0, 1.5, 2.25, 2.5, 2.75, 3.0, 3.25, 3.5, 3.75, 4.0, 4.25, 4.5, 4.75, 5.0, 5.25, 6.25, 8.0, 10.5, 28.75, -11.25, -7.25, 1.5, 1.75, 2.0, 2.25, 2.5, 2.75, 3.0, 3.25, 3.5, 3.75, 4.0, 4.25, 4.75, 5.0, 5.25, 5.5, 5.75, 6.0, 6.25, 6.5, 7.0, 7.25, 7.5, 7.75, 14.25, 1.75, 2.0, 2.5, 3.25, 3.75, 4.0, 5.75, 6.0, 6.25, 6.5, 6.75, 7.5, 9.25, 13.0, 13.25, 14.0, 1.75, 2.0, 2.5, 3.0, 3.25, 3.5, 6.0, 8.0, 8.25, 9.25, 10.25, 13.5, 13.75, -1.75, -1.5, -1.25, 3.25, 3.5, 4.0, 7.0, 8.0, 9.0, 13.0, -9.5, -5.0, -4.5, -4.25, -4.0, -3.75, -2.0, -1.75, -1.5, -1.25, -1.0, -0.75, -0.5, -0.25, 0.0, 0.25, 6.0, 7.5, 8.75, 9.5, 10.25, 12.25, 12.5, -5.5, -5.25, -5.0, -4.75, -4.5, -4.0, -3.75, -3.5, -2.0, -1.75, -1.0, -0.25, 0.25, 1.0, 1.25, 1.5, 7.5, 10.5, 10.75, -6.75, -6.5, -6.25, -6.0, -5.75, -5.5, 1.0, 1.25, 5.75, 10.5, -7.5, -7.25, -7.0, -6.75, -6.5, -3.5, -3.25, 1.25, 10.25, -7.0, -6.75, -3.5, 9.0, -4.0, -4.25, 17.25, 17.0, 17.0, 3.0, 3.25, 16.5, 16.5, 16.75, 3.0, 13.0, 13.25, 13.5, 13.75, 14.0, 14.25, 14.5, 14.75, 15.0, 15.25, 15.25, 15.5, 15.75, 16.0, 16.25, 16.5, 4.75, 5.0, 10.25, 16.75, 17.0, 17.25, 4.25, 4.5, 4.75, 5.0, 5.25, 5.5, 5.75, 6.0, 6.25, 6.5, 10.25, 4.25, 6.5, 6.75, 7.0, 7.25, 7.5, 7.75, 8.0, 10.0, 10.0]}, {"Y"=[-1.75], "Y"=[8.75]}, {"Y"=[-23.75, -23.5, -23.5, -22.0, -21.75, -17.5, -13.0, -13.0, -12.75, -12.5, -12.25, -11.5, -10.75, -10.75, -10.5, -10.5, -10.5, -10.5, -10.25, -10.25, -10.25, -10.0, -9.75, -9.5, -9.5, -9.5, -9.25, -9.25, -9.0, -9.0, -9.0, -9.0, -8.75, -8.75, -8.75, -8.75, -8.75, -8.75, -8.75, -8.75, -8.75, -8.5, -8.5, -8.5, -8.5, -8.5, -8.5, -8.5, -8.25, -8.25, -8.25, -8.25, -8.25, -8.25, -8.25, -8.25, -8.25, -8.25, -8.25, -8.0, -8.0, -8.0, -8.0, -7.75, -7.75, -7.75, -7.75, -7.75, -7.75, -7.75, -7.75, -7.75, -7.5, -7.5, -7.5, -7.5, -7.5, -7.5, -7.5, -7.5, -7.5, -7.5, -7.5, -7.5, -7.25, -7.25, -7.25, -7.25, -7.25, -7.25, -7.25, -7.25, -7.25, -7.25, -7.25, -7.25, -7.25, -7.25, -7.0, -7.0, -7.0, -7.0, -7.0, -7.0, -7.0, -7.0, -7.0, -7.0, -6.75, -6.75, -6.75, -6.75, -6.75, -6.75, -6.75, -6.75, -6.75, -6.75, -6.75, -6.5, -6.5, -6.5, -6.5, -6.5, -6.25, -6.25, -6.25, -6.25, -6.25, -6.25, -6.25, -6.25, -6.25, -6.25, -6.25, -6.25, -6.0, -6.0, -5.75, -5.75, -5.75, -5.75, -5.75, -5.75, -5.75, -5.75, -5.75, -5.75, -5.75, -5.75, -5.75, -5.75, -5.75, -2.25, -2.25, -2.25, -2.25, -2.25, -2.25, -2.25, -2.25, -2.25, -2.25, -2.25, -2.25, -2.25, -2.25, -2.25, -2.25, -2.25, -2.25, -2.0, -2.0, -2.0, -2.0, -2.0, -2.0, -2.0, -2.0, -2.0, -2.0, -2.0, -2.0, -2.0, -2.0, -2.0, -2.0, -2.0, -2.0, -2.0, -2.0, -2.0, -2.0, -2.0, -2.0, -1.75, -1.75, -1.75, -1.75, -1.75, -1.75, -1.75, -1.75, -1.75, -1.75, -1.75, -1.75, -1.75, -1.75, -1.75, -1.75, -1.75, -1.5, -1.5, -1.5, -1.5, -1.5, -1.5, -1.5, -1.5, -1.5, -1.5, -1.5, -1.5, -1.5, -1.25, -1.25, 1.75, 1.75, 1.75, 1.75, 1.75, 1.75, 1.75, 1.75, 1.75, 1.75, 1.75, 1.75, 1.75, 2.0, 2.0, 2.0, 2.0, 2.0, 2.0, 2.0, 2.0, 2.0, 2.0, 2.25, 2.25, 2.5, 2.5, 2.5, 2.5, 2.5, 2.5, 2.75, 2.75, 2.75, 2.75, 2.75, 2.75, 2.75, 2.75, 2.75, 3.0, 3.0, 3.0, 3.0, 3.0, 3.0, 3.0, 3.0, 3.25, 3.25, 3.25, 3.25, 3.25, 3.25, 3.25, 3.25, 3.5, 3.5, 3.5, 3.5, 3.5, 3.75, 4.0, 4.0, 4.0, 4.0, 4.25, 4.25, 4.25, 4.5, 4.5, 4.5, 4.5, 4.75, 4.75, 4.75, 5.0, 5.0, 5.5, 6.5, 7.0, 7.0, 7.25, 7.5, 7.5, 7.75, 7.75, 8.0, 8.25, 8.5, 8.75, 8.75, 10.5, 10.75, 11.0, 11.0, 11.0, 11.0, 11.0, 11.0, 11.25, 11.25, 11.25, 11.25, 11.25, 11.25, 11.25, 11.25, 11.5, 11.5, 11.5, 11.5, 11.5, 11.5, 11.5, 11.5, 11.5, 11.5, 11.5, 11.5, 11.75, 11.75, 11.75, 11.75, 11.75, 12.0, 12.0, 12.0, 12.0, 12.0, 12.0, 12.0, 12.25, 12.25, 12.5, 12.75, 13.5, 13.5, 13.5, 13.5, 13.5, -2.25, -2.25, -1.75], "Y"=[24.75, 24.75, 25.0, 24.75, 24.75, 15.25, 1.0, 4.5, 20.0, 19.75, 0.5, 14.25, 14.25, 14.5, 6.0, 14.5, 14.75, 15.5, 14.75, 15.0, 15.25, 9.5, 3.5, -3.0, 3.0, 3.25, 8.25, 16.75, 0.5, 1.5, 8.25, 12.25, 1.0, 1.25, 1.5, 2.0, 2.25, 6.0, 8.0, 8.5, 12.75, -11.5, -5.75, 1.0, 2.25, 3.0, 9.0, 12.75, -13.25, -11.0, -4.5, -1.25, 3.0, 3.25, 4.0, 6.5, 8.75, 9.0, 9.25, -15.0, 8.75, 9.0, 9.25, -13.5, -8.0, -6.25, -3.0, -2.75, 1.75, 2.0, 2.25, 9.75, -11.5, -4.5, -2.75, -1.0, -0.75, 0.0, 2.0, 2.75, 3.0, 7.0, 7.25, 7.5, -14.25, -11.5, -8.5, -8.0, -4.75, -4.25, -3.25, -3.0, -0.75, 0.25, 0.75, 2.75, 3.0, 7.75, -14.75, -14.5, -11.5, -8.25, -1.5, -1.25, 1.0, 8.0, 8.25, 10.5, -11.75, 0.25, 0.5, 0.75, 1.5, 2.0, 2.25, 2.5, 6.5, 6.75, 8.25, -19.0, 0.25, 0.5, 0.75, 6.25, -5.75, -2.5, -0.25, 0.0, 0.25, 0.5, 0.75, 1.0, 1.25, 1.5, 1.75, 2.0, 5.0, 6.25, -12.25, -10.0, -5.25, -4.25, -4.0, -3.0, -0.75, -0.5, -0.25, 2.0, 2.25, 2.5, 3.75, 4.0, 5.0, -3.25, -3.0, -2.5, -2.25, 3.0, 3.25, 3.5, 3.75, 4.0, 4.25, 4.5, 4.75, 5.0, 5.25, 5.5, 6.0, 6.5, 7.25, -12.75, -10.75, -9.25, -9.0, -8.0, -7.0, -6.25, -5.5, -5.0, -4.5, -4.0, -3.5, -3.25, -3.0, -2.75, -2.5, -2.25, 3.0, 3.25, 3.5, 3.75, 4.25, 4.5, 15.25, -15.5, -12.75, -10.75, 3.5, 3.75, 4.0, 4.25, 4.5, 4.75, 5.0, 5.25, 5.75, 6.25, 6.75, 7.25, 8.0, 15.25, -12.75, -10.75, -9.25, -8.0, -7.0, -6.25, -5.75, -5.25, -5.0, -4.5, -4.25, -3.75, -3.5, -15.75, -12.75, 3.25, 3.5, 3.75, 4.0, 4.25, 4.5, 4.75, 5.0, 5.25, 5.75, 6.25, 6.75, 7.25, -13.0, -4.5, -4.25, -3.75, 6.0, 6.25, 6.75, 7.25, 8.0, 8.75, 3.75, 10.0, 4.25, 4.5, 4.75, 6.0, 7.75, 11.25, -7.0, -6.0, -5.25, 7.5, 7.75, 8.5, 9.5, 9.75, 12.75, -12.5, -12.25, -6.75, -6.0, -5.75, 8.25, 8.5, 9.25, -10.5, -8.75, -8.5, 9.0, 10.25, 10.5, 12.5, 15.25, -15.5, -15.0, -10.5, -8.75, 10.5, -3.25, -12.5, -12.25, -10.0, -6.25, -8.0, -5.5, 2.25, -9.75, -8.0, -6.25, -4.75, -12.75, -5.25, -5.0, -12.5, 1.5, 1.5, 3.75, 1.25, 5.5, 5.5, 3.5, 5.75, 1.75, 3.5, 3.5, 8.0, 3.75, -1.5, 8.25, 3.5, 3.0, 2.5, 4.0, 4.25, 4.75, 5.25, 9.25, -5.5, -3.75, -2.0, 1.75, 3.25, 3.5, 8.5, 10.75, -7.5, -5.25, 1.25, 3.0, 3.25, 3.5, 8.0, 8.5, 9.5, 9.75, 10.25, 10.5, -7.5, -5.25, 1.75, 2.0, 7.5, -4.5, -4.25, -3.75, 6.75, 8.0, 13.75, 14.0, -3.5, 13.5, 12.25, 12.5, -0.75, -0.5, -0.25, 0.0, 0.25, 8.75, 12.75, 8.75]}, {"Y"=[0.85, 0.95, 0.95, 0.6, 0.6, 0.85, 0.85, -0.85, -0.85, -0.95, -0.95, -0.6, -0.6, -0.85, -0.6, -0.6, -0.85, -0.85, 0.85, 0.85], "Y"=[-0.6, -0.6, -1.4, -1.4, -0.6, -0.6, 2.4, 2.4, -0.6, -0.6, -1.4, -1.4, -0.6, -0.6, -0.6, -1.4, -1.4, -1.6, -1.6, -1.4]}]
  in  "Make WPT":bool
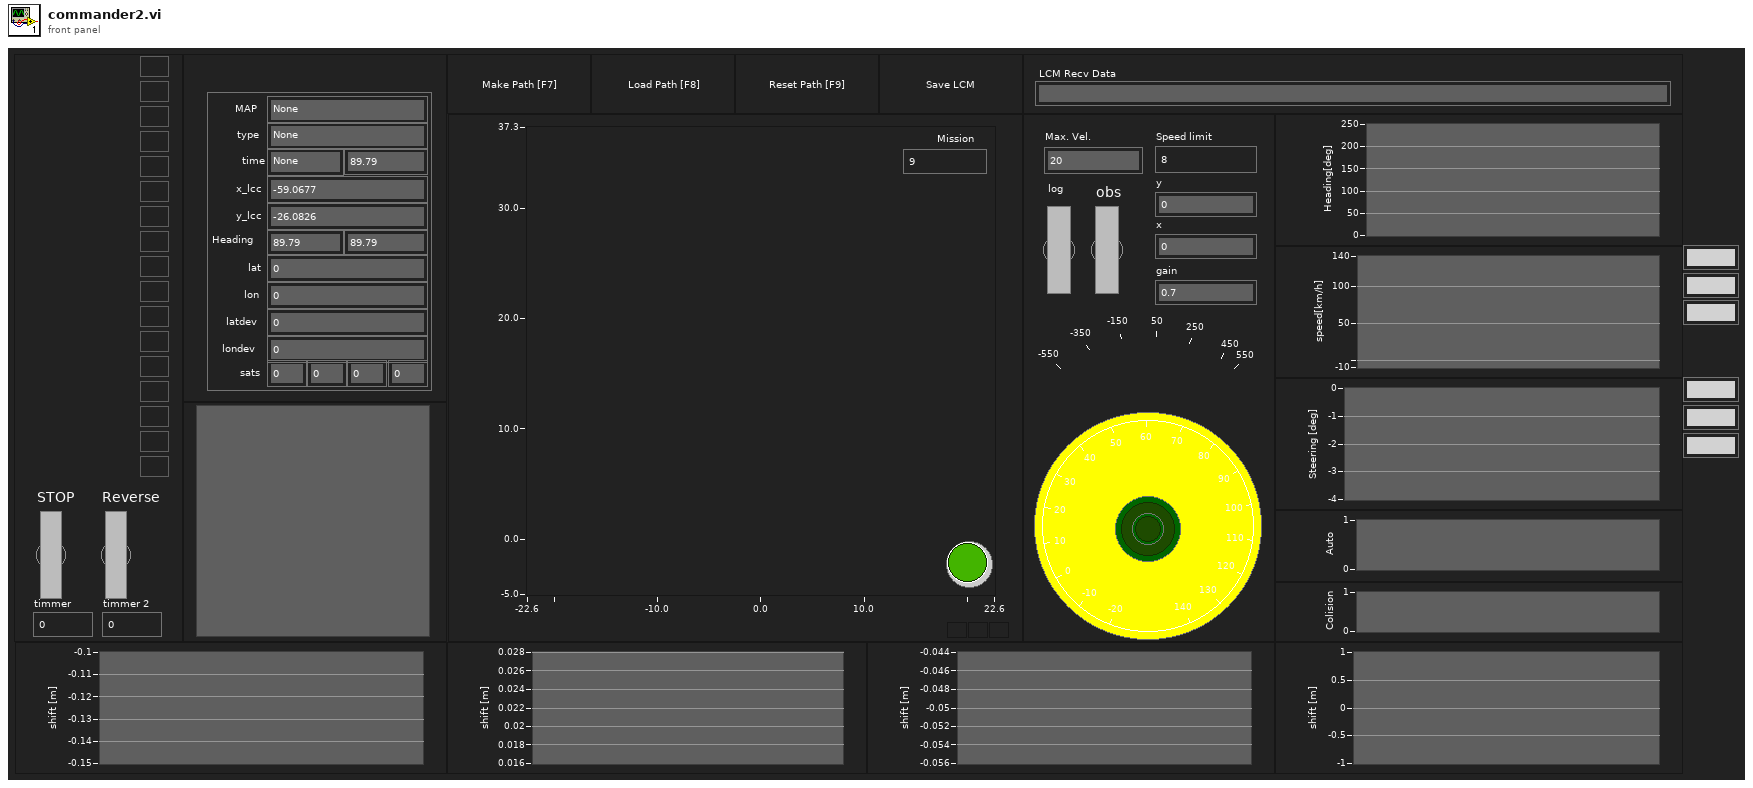
[diagram p1: front panel]
types:
  T1 = cluster{"type":string, "x_lcc":dbl, "y_lcc":dbl, "latdev":sgl, "londev":sgl, "sats":u8, "gps_l1_ranges":u8, "gps_l1_mask_ranges":u8, "gps_l2_mask_ranges":u8, "Heading":dbl, "lon":sgl, "lat":sgl, "time":string, "hgps":dbl, "lag":dbl, "MAP":string}
  T2 = cluster{"Steer_input":dbl, "Steer_output":dbl, "handle":dbl}
  T3 = cluster{"VS_des":dbl, "VS_can":dbl, "VS_des":dbl}
  T4 = cluster{"X":cluster{"idx":i32, "x":dbl, "y":dbl, "h":dbl, "x_path":dbl}}[]
  T5 = cluster{"idx":i32, "x":dbl, "y":dbl, "h":dbl, "x_path":dbl}
  T6 = cluster{"idx":i32, "x":dbl, "y":dbl, "hp":dbl, "x_path":dbl}
  T7 = cluster{"GPSTime":dbl, "attitude[2]":dbl, "lcc[0]":dbl, "lcc[1]":dbl, "heading_GPS":dbl}
  T8 = cluster{"Steer_input":dbl, "Steer_output":dbl, "VS_des":dbl, "VS_can":dbl, "heading":dbl, "auto":bool, "run":bool, "x":dbl, "y":dbl}
  T9 = cluster{"c_idx":i32, "xc":dbl, "yc":dbl, "hc":dbl, "xc_path":dbl}
  T10 = cluster{"hash":i64, "sys time":i64, "dt":dbl, "x":dbl, "y":dbl, "speed":dbl, "heading":dbl, "yaw_rate":dbl}
  T11 = cluster{"Minimum":dbl, "Minimum":dbl, "Minimum":dbl, "Minimum":dbl, "Minimum":dbl}
  T12 = cluster{"X":cluster{"c_idx":i32, "xc":dbl, "yc":dbl, "hc":dbl, "xc_path":dbl}}[]
  T13 = cluster{"x":cluster{"idx":i32, "x":dbl, "y":dbl, "h":dbl, "x_path":dbl}}[]
  T14 = cluster{"hash":i64, "sys time":i64, "time":dbl, "x":dbl, "y":dbl, "h":dbl, "numSV":i32, "postype":i32, "lag":i32, "hordev":dbl, "lat":dbl, "lon":dbl, "hgt":dbl, "map_idx":i32}
  T15 = typedef "NI_Matrix.lvlib/RealMatrix.ctl" = dbl[][]
  T16 = cluster{"idx":bool, "x":bool, "y":bool, "h":bool, "x_path":bool}
  T17 = cluster{"idx":dbl, "x":dbl, "y":dbl, "h":dbl, "x_path":dbl}
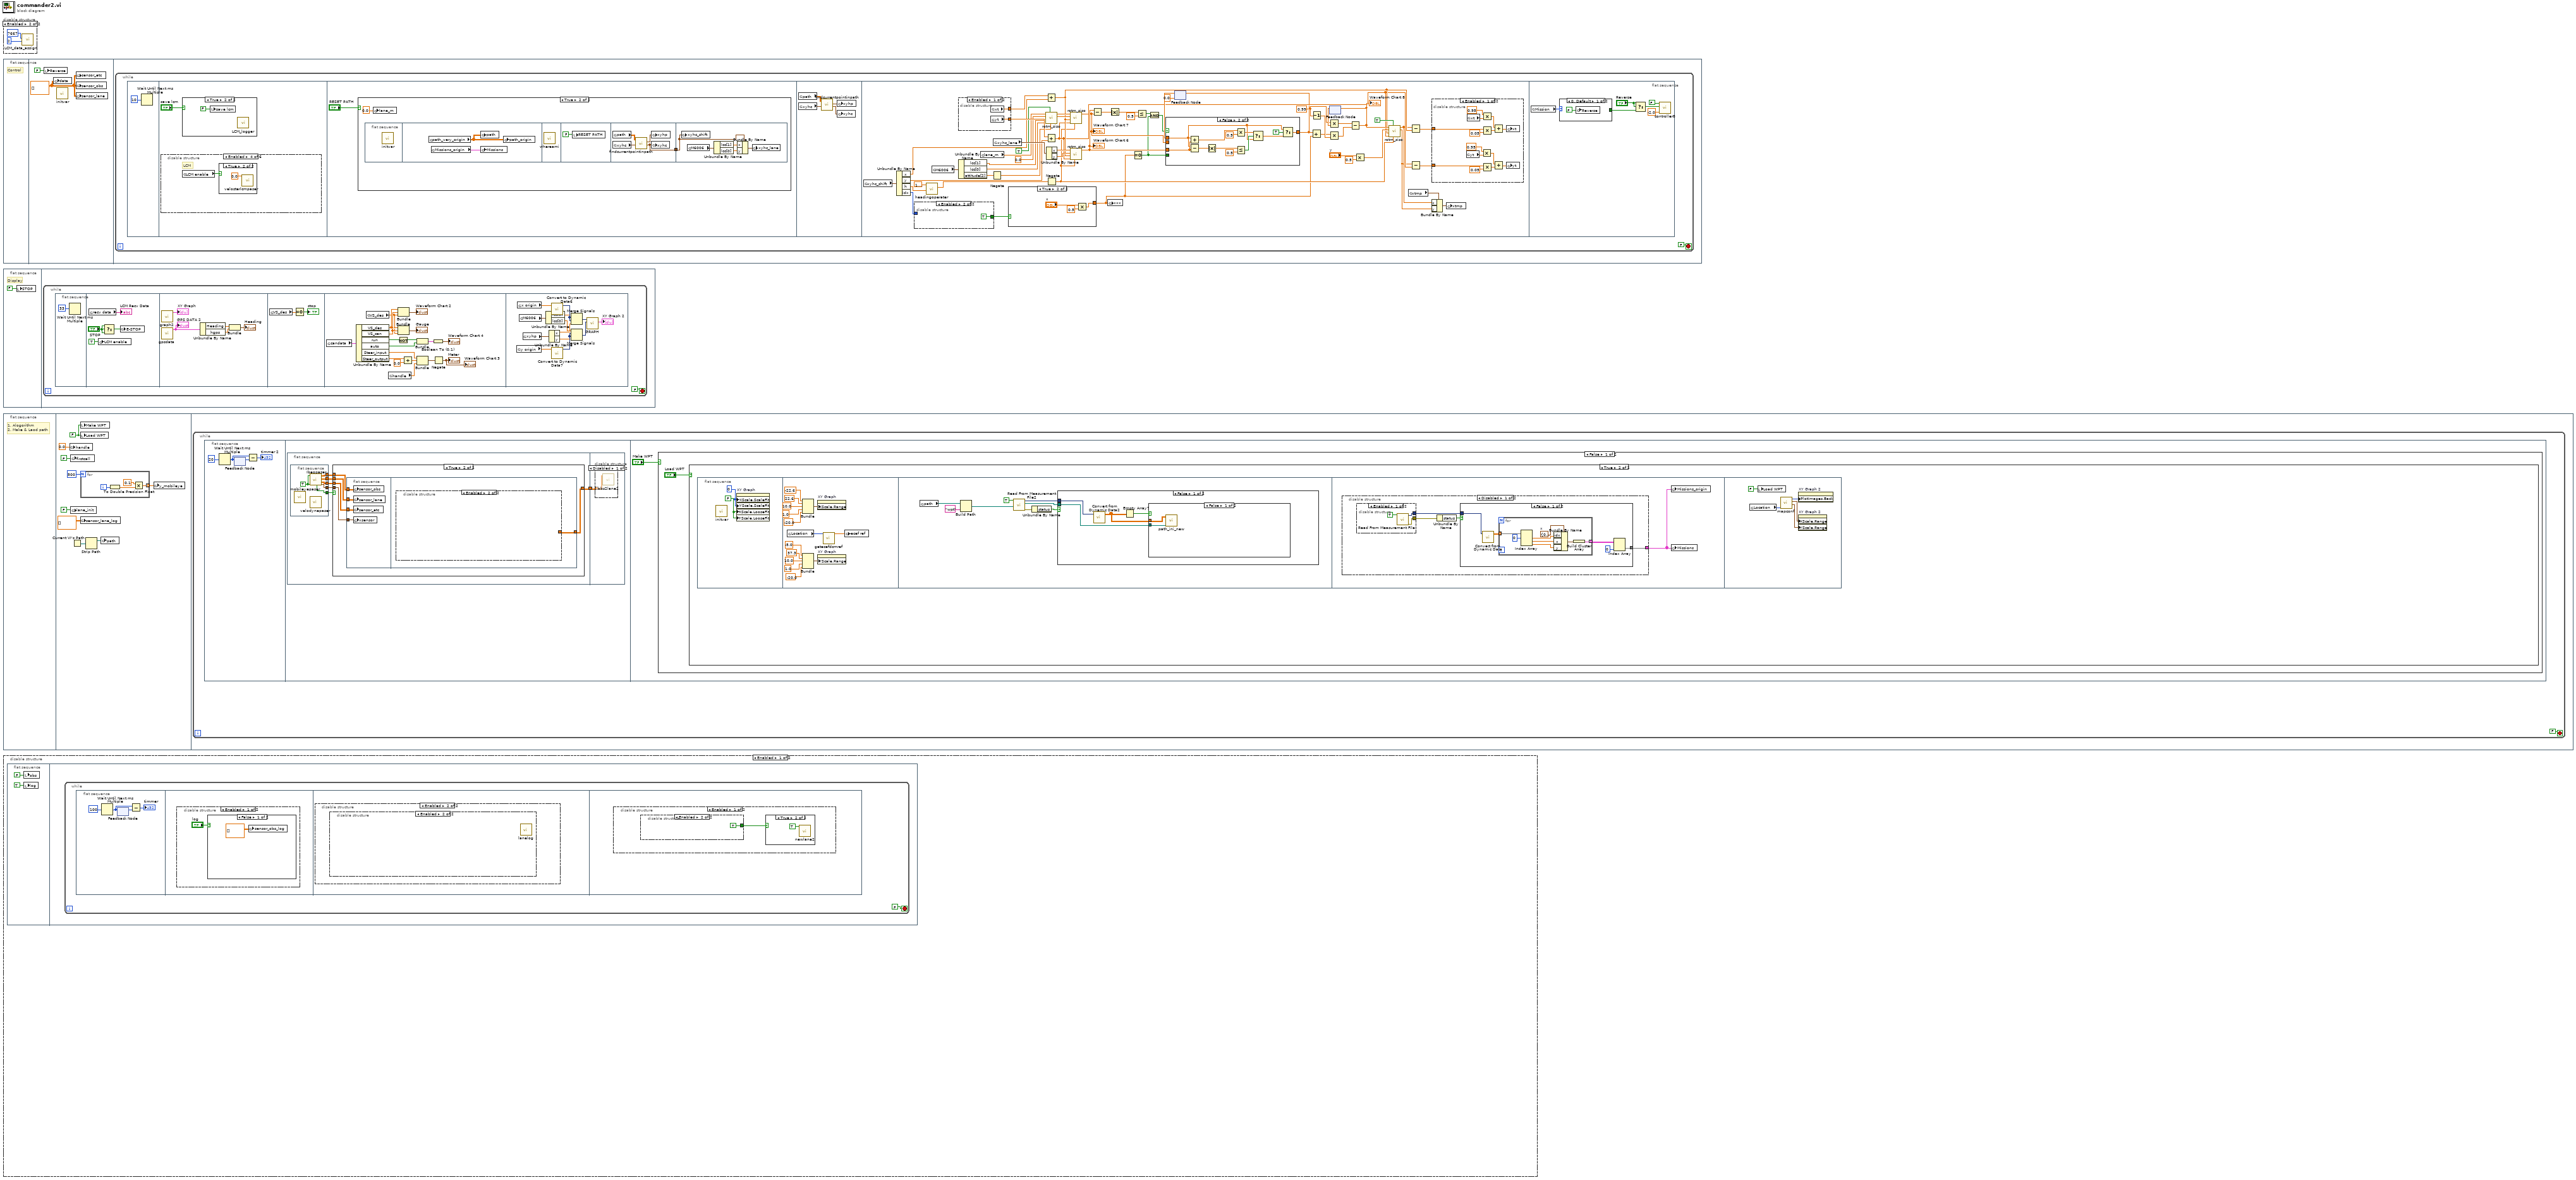
[diagram p0: block diagram]
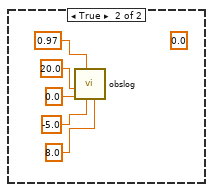
[diagram p2: hidden frame]
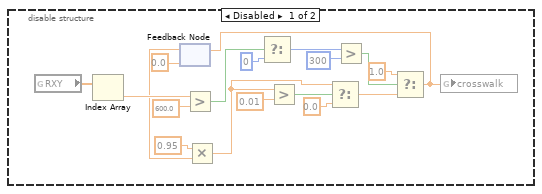
[diagram p5: hidden frame]
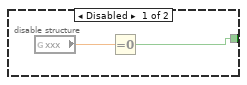
[diagram p6: hidden frame]
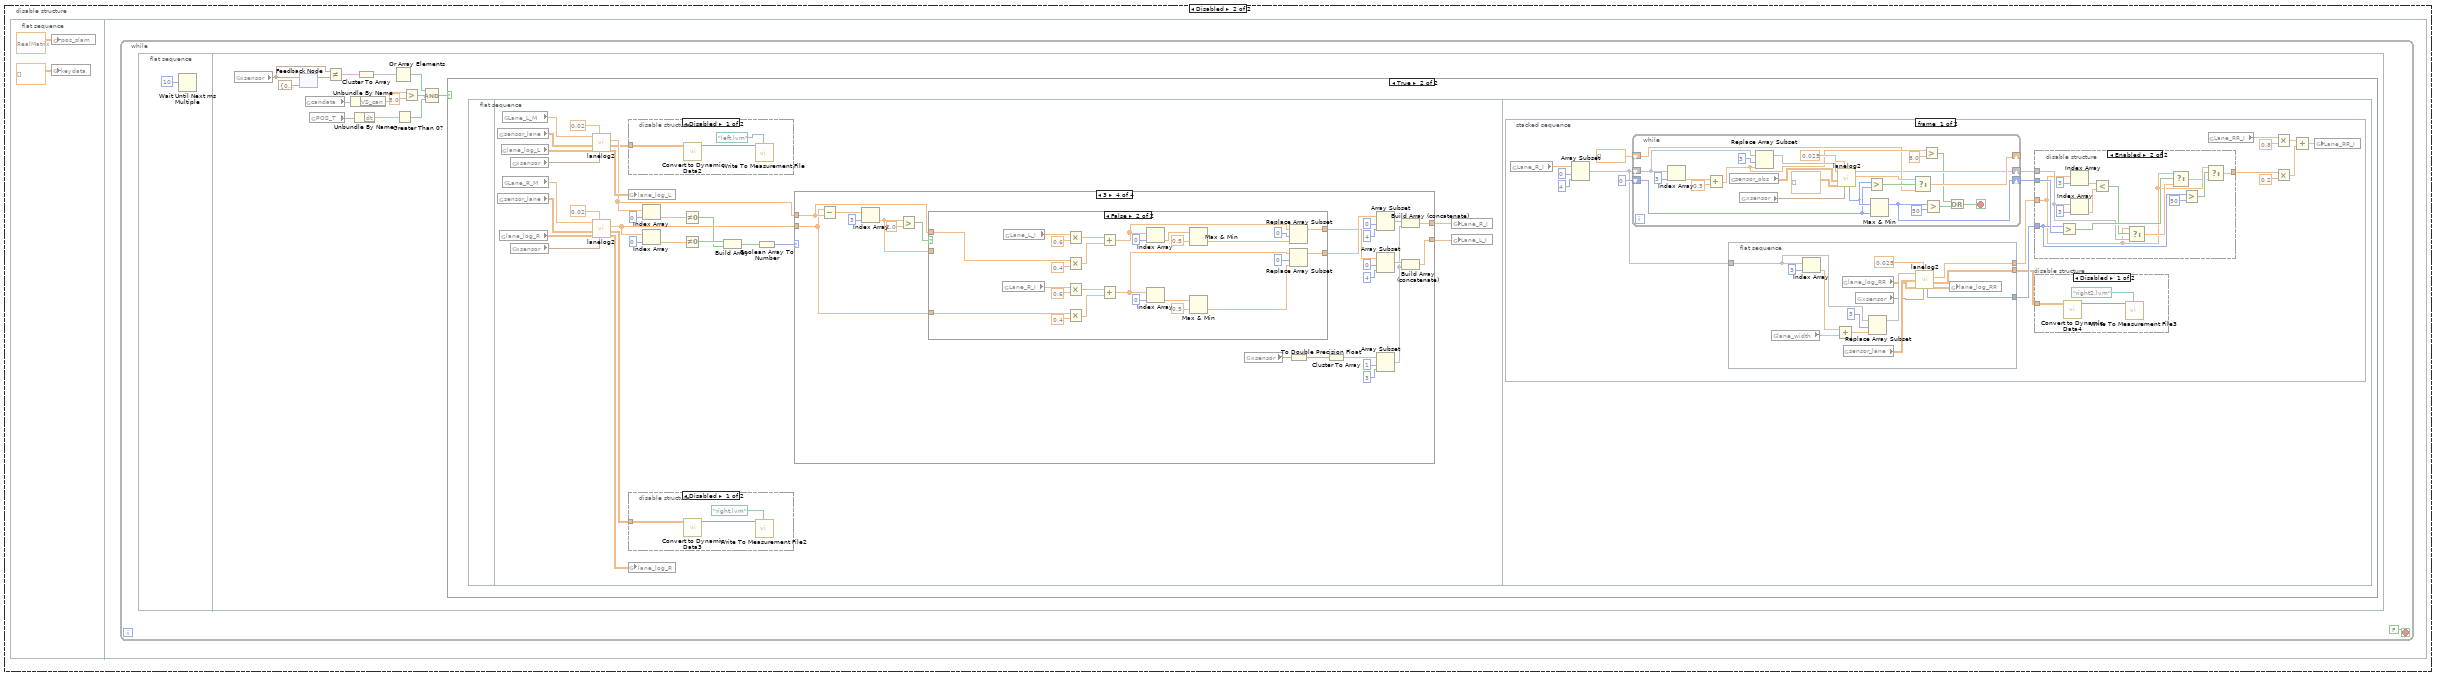
[diagram p9: hidden frame]
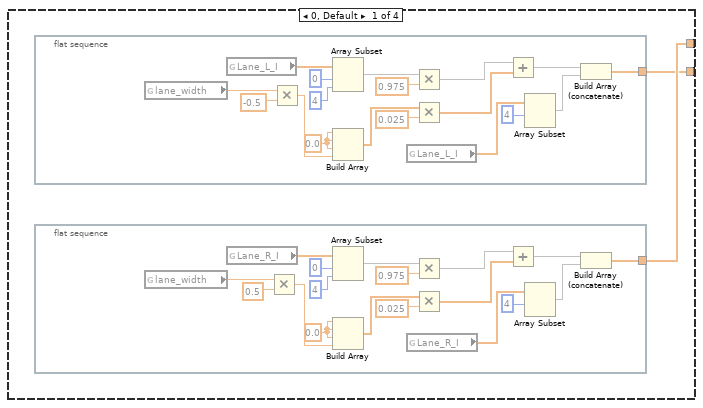
[diagram p13: hidden frame]
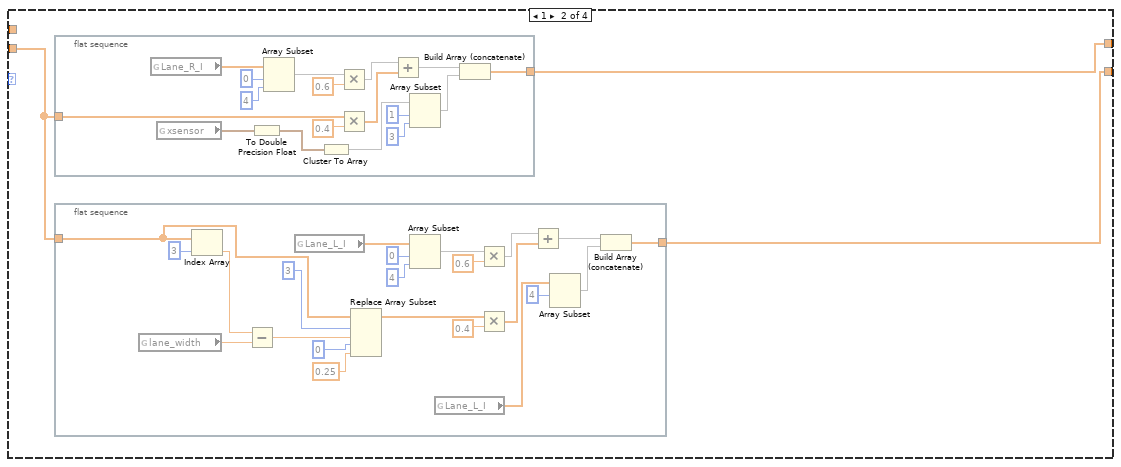
[diagram p14: hidden frame]
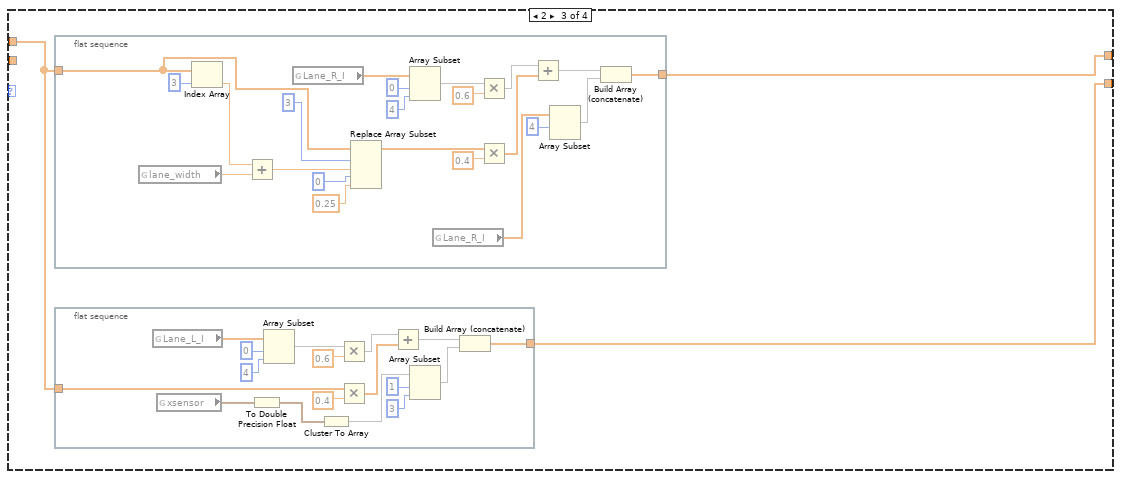
[diagram p15: hidden frame]
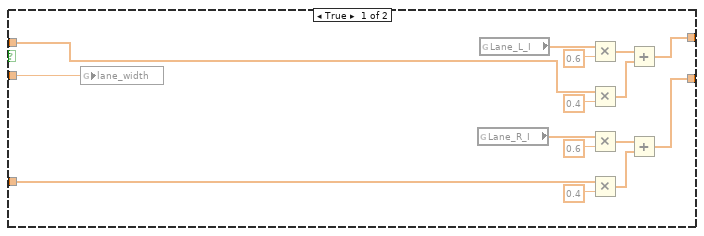
[diagram p16: hidden frame]
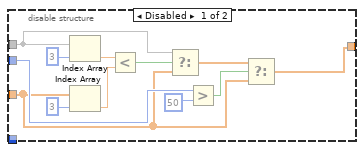
[diagram p18: hidden frame]
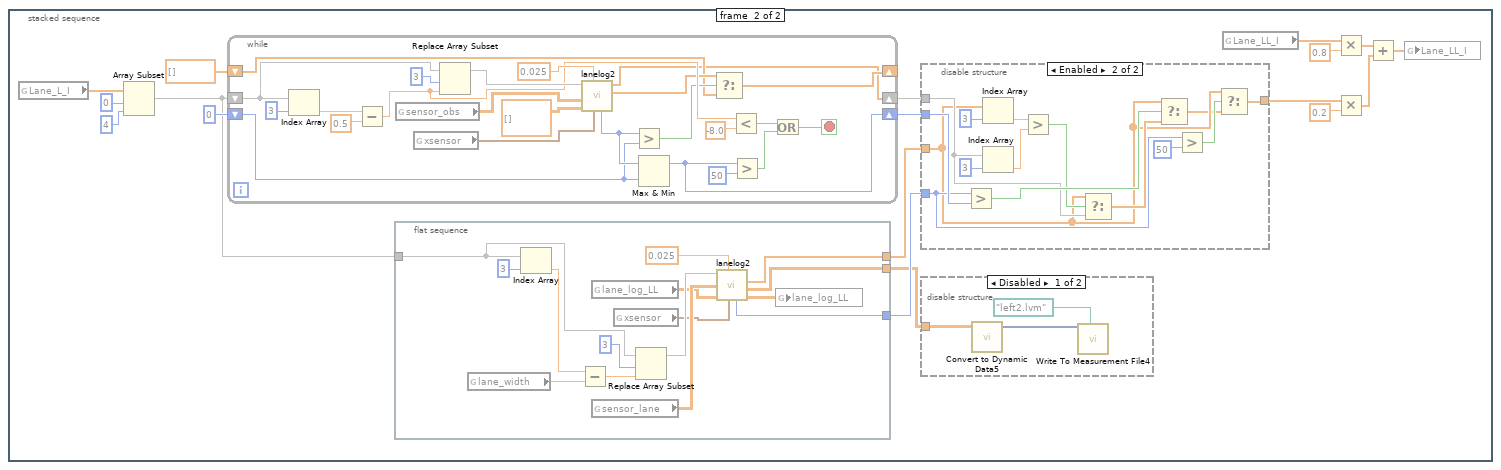
[diagram p19: hidden frame]
diagram:
  n1 = disable-structure shown="Enabled" {
    frame Disabled {
      n2 = call "comm.vi"() -> ()  [unwired: 12 in]
    }
    frame Enabled {
      n3 = call "LCM_data_assign.vi"("time-to-live"=u16 2, "port"=u16 7667) -> ()  [unwired: 10 in]
    }
  }
  n4 = flat-sequence {
    frame #0 {
      # "Control"
    }
    frame #1 {
      w3 = dbl[][] [] ("sensor_car")
      n5 = local write "Reverse"(FALSE ("STOP Signal")) -> ()
      n6 = global write "G_SEN.vi" "data"(w3) -> ()
      n7 = call "initvar.vi"() -> ()  [unwired: 12 in]
      n8 = global write "G_SEN.vi" "sensor_etc"(w3) -> ()
      n9 = global write "G_SEN.vi" "sensor_obs"(w3) -> ()
      n10 = global write "G_SEN.vi" "sensor_lane"(w3) -> ()
    }
    frame #2 {
      n11 = while {
        stop <- FALSE ("Boolean") stop-if-true
        n12 = flat-sequence {
          frame #0 {
            n13 = Wait Until Next ms Multiple(millisecond multiple=u32 10 ("milliseconds to wait")) -> ()  [unwired: 1 out]
          }
          frame #1 {
            n14 = disable-structure shown="Enabled" {
              frame Disabled {
                n15 = global read "G_DATA.vi" "Load data"() -> (w9:bool)
                n16 = case shown="False" w9 {
                  frame False {
                    # "soul"
                    n17 = call "soulpaser.vi"("rionav?"=FALSE) -> ()  [unwired: 11 in]
                  }
                  frame True {
                  }
                }
              }
              frame Disabled {
                n18 = global read "G_DATA.vi" "Load data"() -> (w11:bool)
                n19 = case shown="False" w11 {
                  frame False {
                    # "veloster"
                    n20 = call "velosterpaser.vi"("x"=0.0) -> ()  [unwired: 11 in]
                  }
                  frame True {
                  }
                }
              }
              frame Disabled {
                n21 = global read "G_DATA.vi" "Load data"() -> (w13:bool)
                n22 = case shown="True" w13 {
                  frame False {
                    # "webot"
                    n23 = call "webot.vi"() -> ()  [unwired: 12 in]
                  }
                  frame True {
                  }
                }
              }
              frame Enabled {
                # "LCM"
                n24 = global read "G_LCM.vi" "LCM enable"() -> (w14:bool)
                n25 = case shown="True" w14 {
                  frame False {
                  }
                  frame True {
                    n26 = call "velosterlcmpaser.vi"("x"=0.0) -> ()  [unwired: 11 in]
                  }
                }
              }
              frame Disabled {
              }
              frame Disabled {
                # "RCcar"
                n27 = global read "G_DATA.vi" "Load data"() -> (w16:bool)
                n28 = case shown="True" w16 {
                  frame False {
                  }
                  frame True {
                    n29 = global read "G_VEH.vi" "VS_des"() -> (w17:dbl)
                    n30 = global read "G_VEH.vi" "handle"() -> (w18:dbl)
                    n31 = shared-variable "NI-sbRIO9606-01866155\\sharedvari.lvlib\\vs_des"(w17) -> ()  [unwired: 1 in, 1 out]
                    n32 = shared-variable "NI-sbRIO9606-01866155\\sharedvari.lvlib\\steer_input"(w18) -> ()  [unwired: 1 in, 1 out]
                  }
                }
              }
            }
            n33 = case shown="True" "save lcm" {
              frame False {
              }
              frame True {
                n34 = local write "save lcm"(FALSE ("save lcm")) -> ()
                n35 = call "LCM_logger.vi"() -> ()  [unwired: 12 in]
              }
            }
          }
          frame #2 {
            n36 = case shown="True" "RESET PATH" {
              frame False {
                n37 = disable-structure shown="Enabled" {
                  frame Enabled {
                  }
                  frame Disabled {
                    n38 = call "commpaser.vi"("y_shift"=1.7000000000000006, "large map"=TRUE) -> ("lane"=w26:dbl[][], "obs"=w27:dbl[][], "size(s)"=w31:i32, "etc"=w24:dbl[][])  [unwired: 5 in, 1 out]
                    n39 = call "Ibeopaser.vi"() -> ("etc"=w20:dbl[][], "lane"=w21:dbl[][], "obs"=w22:dbl[][])  [unwired: 7 in, 2 out]
                    n40 = disable-structure shown="Disabled" {
                      disable-tunnel: [w34 w37 w45] -> w28
                      disable-tunnel: w22 -> [w34 _ w44]
                      disable-tunnel: w27 -> [_ w37 w43]
                      disable-tunnel: w26 -> [_ w36 w42]
                      disable-tunnel: w21 -> [w33 _ w41]
                      disable-tunnel: [w33 w36 w40] -> w25
                      disable-tunnel: w24 -> [_ w35 w39]
                      disable-tunnel: [w32 w35 w38] -> w23
                      disable-tunnel: w20 -> [w32 _ _]
                      frame Enabled {
                        # "ibeo"
                      }
                      frame Disabled {
                        # "velodyne"
                      }
                      frame Disabled {
                        # "both"
                        n41 = Build Array (concatenate)(w44, w43) -> (w45:dbl[][])
                        n42 = Build Array (concatenate)(w41, w42) -> (w40:dbl[][])
                        n43 = Build Array (concatenate)(w39) -> (w38:dbl[][])  [unwired: 1 in]
                      }
                    }
                    n44 = global write "G_SEN.vi" "sensor_obs"(w28) -> ()
                    n45 = global write "G_SEN.vi" "sensor_lane"(w25) -> ()
                    n46 = global write "G_SEN.vi" "sensor_etc"(w23) -> ()
                  }
                }
              }
              frame True {
                n47 = flat-sequence {
                  tunnel: [w52] -> w47
                  tunnel: w47 -> [w59]
                  frame #0 {
                    n48 = call "initvar.vi"() -> ()  [unwired: 12 in]
                  }
                  frame #1 {
                    n49 = global read "G_PATH.vi" "path_very_origin"() -> (w49:dbl[][])
                    n50 = global read "G_PATH.vi" "Missions_origin"() -> (w48:T4)
                    n51 = global write "G_PATH.vi" "path"(w49) -> ()
                    n52 = global write "G_PATH.vi" "Missions"(w48) -> ()
                    n53 = global write "G_PATH.vi" "path_origin"(w49) -> ()
                  }
                  frame #2 {
                    n54 = call "whereami.vi"() -> ()  [unwired: 12 in]
                  }
                  frame #3 {
                    n55 = local write "RESET PATH"(FALSE ("RESET PATH")) -> ()
                  }
                  frame #4 {
                    n56 = global read "G_PATH.vi" "path"() -> (w51:dbl[][])
                    n57 = global read "G_VEH.vi" "xyhc"() -> (w53:T5)
                    n58 = call "findcurrentpointinpath.vi"("xyhc_in"=w53, "path_updated"=w51) -> ("xyhc_out"=w52:T5, "xyhp"=w54:T6)  [unwired: 8 in]
                    n59 = global write "G_VEH.vi" "xyhp"(w54) -> ()
                    n60 = global write "G_VEH.vi" "xyhc"(w52) -> ()
                  }
                  frame #5 {
                    n61 = global write "G_VEH.vi" "xyhc_shift"(w59) -> ()
                    n62 = global read "G_NAV.vi" "M6006"() -> (w57:T7)
                    n63 = Unbundle By Name(w57) -> ("lcc[1]"=w56:dbl, "lcc[0]"=w55:dbl)
                    n64 = Bundle By Name(cluster=w59, "x"=w56, "y"=w55) -> (w58:T5)
                    n65 = global write "G_VEH.vi" "xyhc_lane"(w58) -> ()
                  }
                }
                n66 = global write "G_SEN.vi" "lane_m"(0.0 ("lane_m")) -> ()
              }
            }
          }
          frame #3 {
            n67 = global read "G_PATH.vi" "path"() -> (w60:dbl[][])
            n68 = global read "G_VEH.vi" "xyhc"() -> (w63:T5)
            n69 = call "findcurrentpointinpath.vi"("xyhc_in"=w63, "path_updated"=w60) -> ("xyhc_out"=w61:T5, "xyhp"=w62:T6)  [unwired: 8 in]
            n70 = global write "G_VEH.vi" "xyhp"(w62) -> ()
            n71 = global write "G_VEH.vi" "xyhc"(w61) -> ()
          }
          frame #4 {
            w98 = 0.99 ("x")
            n72 = global read "G_VEH.vi" "xyhc_shift"() -> (w105:T5)
            n73 = Unbundle By Name(w105) -> ("x"=w108:dbl, "y"=w110:dbl, "h"=w114:dbl, "idx"=w104:i32)
            n74 = disable-structure shown="Enabled" {
              disable-tunnel: w104 -> [w120 _]
              disable-tunnel: [w119 TRUE] -> w103
              frame Disabled {
                n75 = feedback #1(w120) -> (w121:i32)
                n76 = feedback-in #1(w120) -> ()
                n77 = Equal?(x=w120, y=w121) -> (x = y?=w119:bool)
              }
              frame Enabled {
              }
            }
            n78 = call "headingoperater.vi"("h1"=w114, "h2"=1.5707963267948966) -> ("h2-h1"=w117:dbl)  [unwired: 8 in, 1 out]
            n79 = global read "G_NAV.vi" "M6006"() -> (w87:T7)
            n80 = disable-structure shown="Enabled" {
              disable-tunnel: [w163 _] -> w109
              disable-tunnel: [w162 _] -> w111
              frame Enabled {
                n81 = global read "G_PATH.vi" "xt"() -> (w163:dbl)
                n82 = global read "G_PATH.vi" "yt"() -> (w162:dbl)
              }
              frame Disabled {
              }
            }
            n83 = Unbundle By Name(w87) -> ("lcc[1]"=w86:dbl, "lcc[0]"=w85:dbl, "attitude[2]"=w84:dbl)
            n84 = global read "G_SEN.vi" "lane_m"() -> (w82:dbl)
            n85 = Negate(x=w84) -> (-x=w83:dbl)
            n86 = global read "G_VEH.vi" "xyhc_lane"() -> (w118:T5)
            n87 = case shown="True" w103 {
              tunnel: [w144 w146] -> w69
              frame False {
                w144 = 0.0 ("x")
                n88 = local write "x"(w144) -> ()
              }
              frame True {
                n89 = Multiply(x="x", y=0.5) -> (x*y=w146:dbl)
              }
            }
            n90 = Add(x=w109, y=w108) -> (x+y=w77:dbl)
            n91 = call "rotm_siso.vi"("angle[rad]"=w83, "reverse"=TRUE, "y0"=w85, "x0"=w86, "y"=0.0, "x"=w82) -> ("y'"=w78:dbl, "x'"=w79:dbl)  [unwired: 4 in]
            n92 = Add(x=w111, y=w110) -> (x+y=w76:dbl)
            n93 = Unbundle By Name(w118) -> ("x"=w107:dbl, "y"=w106:dbl)
            n94 = Negate(x=w117) -> (-x=w75:dbl)
            n95 = call "rotm_siso.vi"("angle[rad]"=w75, "y0"=w76, "x0"=w77, "y"=w78, "x"=w79) -> ("x'"=w74:dbl)  [unwired: 5 in, 1 out]
            "Waveform Chart 7" <- w74
            n96 = call "rotm_siso.vi"("angle[rad]"=w75, "y0"=w76, "x0"=w77, "y"=w106, "x"=w107) -> ("x'"=w91:dbl)  [unwired: 5 in, 1 out]
            "Waveform Chart 6" <- w91
            n97 = Subtract(x=w91, y=w74) -> (x-y=w94:dbl)
            n98 = global write "G_PATH.vi" "xxx"(w69) -> ()
            n99 = Absolute Value(x=w94) -> (abs(x)=w93:dbl)
            n100 = Equal To 0?(x=w69) -> (x = 0?=w66:bool)
            n101 = Less Or Equal?(x=w93, y=0.5) -> (x <= y?=w68:bool)
            n102 = And(x=w68, y=w66) -> (x .and. y?=w67:bool)
            n103 = feedback #2(0.0) -> (w90:dbl)
            n104 = case shown="False" w67 {
              tunnel: w91 -> [w123 w137]
              tunnel: w74 -> [w124 _]
              tunnel: [w125 w133] -> w64
              tunnel: w90 -> [w126 w135]
              tunnel: w66 -> [_ _]
              frame True {
                n105 = Add(x=w124, y=w123) -> (x+y=w131:dbl)
                n106 = Multiply(x=w131, y=0.5) -> (x*y=w127:dbl)
                n107 = Add(x=w126, y=w127) -> (x+y=w128:dbl)
                n108 = Multiply(x=w128, y=0.5) -> (x*y=w125:dbl)
              }
              frame False {
                n109 = Add(x=w135, y=w137) -> (x+y=w139:dbl)
                n110 = Subtract(x=w135, y=w137) -> (x-y=w141:dbl)
                n111 = Absolute Value(x=w141) -> (abs(x)=w142:dbl)
                n112 = Multiply(x=w139, y=0.5) -> (x*y=w138:dbl)
                n113 = Less Or Equal?(x=w142, y=0.5) -> (x <= y?=w136:bool)
                n114 = Select(t=w138, s=w136, f=w135) -> (s? t:f=w134:dbl)
                n115 = Select(t=w135, s=TRUE, f=w134) -> (s? t:f=w133:dbl)
              }
            }
            n116 = feedback-in #2(w64) -> ()
            n117 = Add(x=w64, y=w69) -> (x+y=w65:dbl)
            n118 = Decrement(x=w98) -> (x-1=w97:dbl)
            n119 = Multiply(x=w65, y=w97) -> (x*y=w96:dbl)
            n120 = feedback #3() -> (w99:dbl)  [unwired: 1 in]
            n121 = Multiply(x=w98, y=w99) -> (x*y=w95:dbl)
            n122 = Subtract(x=w95, y=w96) -> (x-y=w88:dbl)
            "Waveform Chart 8" <- w88
            n123 = feedback-in #3(w88) -> ()
            n124 = Multiply(x="y", y=0.5) -> (x*y=w101:dbl)
            n125 = call "rotm_siso.vi"("angle[rad]"=w75, "reverse"=TRUE, "y0"=w76, "x0"=w77, "y"=w101, "x"=w88) -> ("y'"=w70:dbl, "x'"=w71:dbl)  [unwired: 4 in]
            n126 = global read "G_VEH.vi" "xtmp"() -> (w72:T5)
            n127 = Subtract(x=w71, y=w77) -> (x-y=w112:dbl)
            n128 = Subtract(x=w70, y=w76) -> (x-y=w113:dbl)
            n129 = disable-structure shown="Enabled" {
              disable-tunnel: w112 -> [w155 _]
              disable-tunnel: w113 -> [w149 _]
              frame Enabled {
                n130 = global read "G_PATH.vi" "yt"() -> (w152:dbl)
                n131 = global read "G_PATH.vi" "xt"() -> (w159:dbl)
                n132 = Multiply(x=0.95, y=w152) -> (x*y=w151:dbl)
                n133 = Multiply(x=0.95, y=w159) -> (x*y=w157:dbl)
                n134 = Multiply(x=w155, y=0.05 ("x")) -> (x*y=w154:dbl)
                n135 = Multiply(x=w149, y=0.05 ("x")) -> (x*y=w148:dbl)
                n136 = Add(x=w157, y=w154) -> (x+y=w161:dbl)
                n137 = Add(x=w151, y=w148) -> (x+y=w160:dbl)
                n138 = global write "G_PATH.vi" "xt"(w161) -> ()
                n139 = global write "G_PATH.vi" "yt"(w160) -> ()
              }
              frame Disabled {
              }
            }
            n140 = Bundle By Name(cluster=w72, "x"=w71, "y"=w70) -> (w73:T5)
            n141 = global write "G_VEH.vi" "xtmp"(w73) -> ()
          }
          frame #5 {
            n142 = global read "G_PATH.vi" "Mission"() -> (w164:i32)
            n143 = case shown="0, Default" w164 {
              tunnel: [_ w171] -> w168
              frame 0, Default {
                n144 = global write "G_VEH.vi" "Reverse"(FALSE ("Reverse")) -> ()
              }
              frame 9 {
                n145 = global read "G_VEH.vi" "Reverse"() -> (w171:bool)
              }
            }
            n146 = Select(t="Reverse", s="Reverse", f=w168) -> (s? t:f=w167:bool)
            n147 = call "controller8.vi"("Neg max speed"=-2.0, "reverse"=w167, "slowmode"=FALSE ("slow mode")) -> ()  [unwired: 9 in]
          }
        }
      }
    }
  }
  n148 = flat-sequence {
    frame #0 {
      # "Display"
      n149 = local write "STOP"(FALSE ("LCM")) -> ()
    }
    frame #1 {
      n150 = while {
        stop <- FALSE ("exit") stop-if-true
        n151 = flat-sequence {
          frame #0 {
            n152 = Wait Until Next ms Multiple(millisecond multiple=u32 33 ("milliseconds to wait")) -> ()  [unwired: 1 out]
          }
          frame #1 {
            n153 = global read "G_LCM.vi" "recv data"() -> (→"LCM Recv Data":string)
            n154 = global write "G_LCM.vi" "LCM enable"(TRUE ("x")) -> ()
            n155 = Select(t="STOP", s="STOP", f="STOP") -> (s? t:f=w178:bool)
            n156 = global write "G_VEH.vi" "E-STOP"(w178) -> ()
          }
          frame #2 {
            n157 = call "graph2.vi"() -> ("XY Graph"=→"XY Graph":cluster{"Y":dbl[], "Y":dbl[]}[])  [unwired: 10 in, 1 out]
            n158 = call "gpsdata.vi"() -> ("GPS DATA 2"=w181:T1)  [unwired: 11 in]
            "GPS DATA 2" <- w181
            n159 = Unbundle By Name(w181) -> ("Heading"=w183:dbl, "hgps"=w182:dbl)
            n160 = Bundle("Heading"=w183, "hgps"=w182) -> (→"Heading":cluster{"Heading":dbl, "hgps":dbl})  [unwired: 1 in]
          }
          frame #3 {
            n161 = global read "G_VEH.vi" "VS_des"() -> (w185:dbl)
            n162 = Equal To 0?(x=w185) -> (x = 0?=→"stop":bool)
          }
          frame #4 {
            n163 = global read "G_VEH.vi" "candata"() -> (w203:T8)
            n164 = Unbundle By Name(w203) -> ("VS_des"=w195:dbl, "VS_can"=w196:dbl, "run"=w190:bool, "auto"=w191:bool, "Steer_input"=w189:dbl, "Steer_output"=w188:dbl)
            n165 = global read "G_VEH.vi" "VS_des"() -> (w194:dbl)
            n166 = global read "G_VEH.vi" "handle"() -> (w192:dbl)
            n167 = Not(x=w190) -> (.not. x?=w198:bool)
            n168 = Bundle("VS_des"=w195, "VS_can"=w196, "VS_des"=w194) -> (→"Waveform Chart 2":T3)  [unwired: 1 in]
            n169 = Bundle("VS_des"=w195, "VS_can"=w196, "VS_des"=w194) -> (→"Gauge":T3)  [unwired: 1 in]
            n170 = Add(x=w188, y=0.0) -> (x+y=w186:dbl)
            n171 = Bundle(w198, "auto"=w191) -> (w200:cluster{bool, "auto":bool})  [unwired: 1 in]
            n172 = Bundle("Steer_input"=w189, w186, "handle"=w192) -> (w202:cluster{"Steer_input":dbl, dbl, "handle":dbl})  [unwired: 1 in]
            n173 = Boolean To (0,1)(Boolean=w200) -> (0, 1=→"Waveform Chart 4":cluster{i16, "auto":i16})
            n174 = Negate(x=w202) -> (-x=→"Meter" →"Waveform Chart 3":cluster{"Steer_input":dbl, dbl, "handle":dbl})
          }
          frame #5 {
            n175 = global read "G_PATH.vi" "y origin"() -> (w205:dbl[])
            n176 = global read "G_PATH.vi" "x origin"() -> (w206:dbl[])
            n177 = global read "G_NAV.vi" "M6006"() -> (w212:T7)
            n178 = global read "G_VEH.vi" "xyhp"() -> (w204:T5)
            n179 = Unbundle By Name(w212) -> ("lcc[1]"=w213:dbl, "lcc[0]"=w214:dbl)
            n180 = Unbundle By Name(w204) -> ("x"=w208:dbl, "y"=w207:dbl)
            n181 = call "Convert to Dynamic Data6"("Array"=w206) -> ("Dynamic Data Type"=w216:dynamicdata)  [unwired: 3 in]
            n182 = call "Convert to Dynamic Data7"("Array"=w205) -> ("Dynamic Data Type"=w215:dynamicdata)  [unwired: 3 in]
            n183 = Merge Signals(w213, w216, w216, w208) -> (w210:dynamicdata)
            n184 = Merge Signals(w214, w215, w215, w207) -> (w211:dynamicdata)
            n185 = call "GRAPH"("Y Input"=w211, "X Input"=w210) -> ("XY Graph"=→"XY Graph 2":cluster{"Y":dbl[], "Y":dbl[]}[])  [unwired: 3 in, 6 out]
          }
        }
      }
    }
  }
  n186 = flat-sequence {
    frame #0 {
      # "1. Alogorithm\n2. Make & Laod path"
    }
    frame #1 {
      w225 = FALSE ("Make WPT")
      n187 = global write "G_VEH.vi" "handle"(0.0 ("handle")) -> ()
      n188 = global write "G_VEH.vi" "firstcall"(FALSE ("firstcall")) -> ()
      n189 = global write "G_PATH.vi" "lane_init"(FALSE ("lane_init")) -> ()
      n190 = Current VI's Path() -> (path=w221:path)
      n191 = local write "Make WPT"(w225) -> ()
      n192 = local write "Load WPT"(w225) -> ()
      n193 = for {
        N: 500 -> [_]
        tunnel: [w226] -> w217 mode=indexing
        i -> [w229]
        n194 = To Double Precision Float(number=w229) -> (double precision float=w228:dbl)
        n195 = Multiply(x=0.1, y=w228) -> (x*y=w226:dbl)
      }
      n196 = global write "G_SEN.vi" "sensor_lane_log"(dbl[][] [] ("sensor_lane_log")) -> ()
      n197 = Strip Path(path=w221) -> (stripped path=w220:path)  [unwired: 1 out]
      n198 = global write "G_DATA.vi" "path"(w220) -> ()
      n199 = global write "G_SEN.vi" "y_mobileye"(w217) -> ()
    }
    frame #2 {
      n200 = while {
        stop <- FALSE stop-if-true
        n201 = flat-sequence {
          frame #0 {
            n202 = Wait Until Next ms Multiple(millisecond multiple=u32 20 ("milliseconds to wait")) -> (millisecond timer value=w231:u32)
            n203 = feedback #4() -> (w233:u32)  [unwired: 1 in]
            n204 = feedback-in #4(w231) -> ()
            n205 = Subtract(x=w231, y=w233) -> (x-y=→"timmer 2":u32)
          }
          frame #1 {
            n206 = flat-sequence {
              tunnel: [w236] -> w235
              tunnel: w235 -> [w276]
              frame #0 {
                n207 = flat-sequence {
                  tunnel: [w247] -> w241
                  tunnel: [w246] -> w240
                  tunnel: [w245] -> w239
                  tunnel: [w244] -> w238
                  tunnel: [w242] -> w237
                  frame #0 {
                    w243 = TRUE ("Sensor [F12]")
                    n208 = call "mobileyepaser.vi"() -> ()  [unwired: 11 in, 1 out]
                    n209 = call "Ibeopaser.vi"("Hide Transparent"=w243, "Sensor [F12]"=w243) -> ("x_sensor"=w246:T5, "etc"=w244:dbl[][], "lane"=w245:dbl[][], "obs"=w247:dbl[][], "update"=w242:bool)  [unwired: 5 in]
                    n210 = call "velodynepaser.vi"() -> ()  [unwired: 9 in, 3 out]
                  }
                }
                n211 = case shown="True" w237 {
                  tunnel: w241 -> [_ w256]
                  tunnel: w240 -> [_ w255]
                  tunnel: w239 -> [_ w254]
                  tunnel: w238 -> [_ w253]
                  tunnel: [w248 w252] -> w236
                  frame False {
                    n212 = disable-structure shown="Disabled" {
                      disable-tunnel: [w249 _] -> w248
                      frame Disabled {
                        n213 = global read "G_SEN.vi" "sensor_lane_log"() -> (w251:dbl[][])
                        n214 = global read "G_VEH.vi" "xsensor"() -> (w250:T5)
                        n215 = call "sensor_log.vi"("xsensor"=w250, "sensor_log"=w251) -> ("sensor_log_body"=w249:dbl[][])  [unwired: 7 in, 2 out]
                      }
                      frame Enabled {
                      }
                    }
                  }
                  frame True {
                    n216 = flat-sequence {
                      tunnel: w256 -> [w260]
                      tunnel: w255 -> [w259]
                      tunnel: w254 -> [w258]
                      tunnel: w253 -> [w257]
                      tunnel: [w261] -> w252
                      frame #0 {
                        n217 = global write "G_SEN.vi" "sensor_obs"(w260) -> ()
                        n218 = global write "G_SEN.vi" "sensor_lane"(w258) -> ()
                        n219 = global write "G_SEN.vi" "sensor_etc"(w257) -> ()
                        n220 = global write "G_VEH.vi" "xsensor"(w259) -> ()
                      }
                      frame #1 {
                        n221 = disable-structure shown="Enabled" {
                          disable-tunnel: [w270 _] -> w261
                          frame Disabled {
                            n222 = global read "G_VEH.vi" "candata"() -> (w263:T8)
                            n223 = global read "G_LCM.vi" "POS_T"() -> (w267:T10)
                            n224 = Unbundle By Name(w263) -> ("VS_can"=w264:dbl)
                            n225 = Unbundle By Name(w267) -> ("dt"=w268:dbl)
                            n226 = global read "G_SEN.vi" "sensor_lane_log"() -> (w273:dbl[][])
                            n227 = global read "G_SEN.vi" "sensor_lane"() -> (w274:dbl[][])
                            n228 = global read "G_VEH.vi" "xsensor"() -> (w271:T5)
                            n229 = Greater Than 0?(x=w268) -> (x > 0?=w269:bool)
                            n230 = Greater?(x=w264, y=5.0) -> (0:w266:bool)
                            n231 = call "sensor_log.vi"("xsensor"=w271, "sensor_log"=w273, "sensor"=w274) -> ("sensor_log_out"=w272:dbl[][], "sensor_log_body"=w270:dbl[][])  [unwired: 6 in, 1 out]
                            n232 = Compound Arithmetic op=AND(w266, w269) -> (w262:bool)
                            n233 = case shown="True" w262 {
                              tunnel: w272 -> [_ w275]
                              frame False {
                              }
                              frame True {
                                n234 = global write "G_SEN.vi" "sensor_lane_log"(w275) -> ()
                              }
                            }
                          }
                          frame Enabled {
                          }
                        }
                      }
                    }
                  }
                }
              }
              frame #1 {
                n235 = disable-structure shown="Disabled" {
                  disable-tunnel: w276 -> [w277 _]
                  frame Disabled {
                    n236 = call "obs2lane2.vi"("sensors inputs"=w277) -> ()  [unwired: 11 in]
                  }
                  frame Enabled {
                  }
                }
              }
            }
          }
          frame #2 {
            n237 = case shown="False" "Make WPT" {
              frame False {
                n238 = case shown="True" "Load WPT" {
                  frame False {
                    n239 = flat-sequence {
                      tunnel: [w285] -> w280
                      tunnel: w280 -> [w380]
                      frame #0 {
                        n240 = Select(t=9 ("Mission"), s=FALSE ("Parking mode"), f=0 ("Mission")) -> (s? t:f=w281:i32)
                        n241 = global write "G_PATH.vi" "Mission"(w281) -> ()
                      }
                      frame #1 {
                        n242 = disable-structure shown="Enabled" {
                          disable-tunnel: [_ w327] -> w285
                          frame Enabled {
                            n243 = global read "G_PATH.vi" "lane_width"() -> (w315:dbl)
                            n244 = Multiply(x=w315, y=0.5) -> (x*y=w310:dbl)
                            n245 = Add(x=w310, y=0.25) -> (x+y=w308:dbl)
                            n246 = Decrement(x=w308) -> (x-1=w305:dbl)
                            n247 = Multiply(x=w305, y=10.0) -> (x*y=w303:dbl)
                            n248 = global read "G_VEH.vi" "handle"() -> (w317:dbl)
                            n249 = Max & Min(x=0.0, y=w303) -> (max(x,y)=w312:dbl)  [unwired: 1 out]
                            n250 = Negate(x=w312) -> (-x=w311:dbl)
                            n251 = Multiply(x=0.5, y=w317) -> (x*y=w321:dbl)
                            n252 = feedback #5() -> (w291:dbl)  [unwired: 1 in]
                            "Waveform Chart 5" <- w291
                            n253 = call "findmovablepath13.vi"("x"=w291) -> ("shift"=w287:dbl, "theta handle"=w300:dbl)  [unwired: 9 in]
                            n254 = disable-structure shown="Enabled" {
                              disable-tunnel: w300 -> [w323 w326]
                              disable-tunnel: [w322 w325] -> w299
                              frame Disabled {
                                n255 = feedback #6(w323) -> (w322:dbl)
                                n256 = feedback-in #6(w323) -> ()
                              }
                              frame Enabled {
                                n257 = Multiply(x=w326, y="gain") -> (x*y=w325:dbl)
                              }
                            }
                            n258 = Equal To 0?(x=w287) -> (x = 0?=→"x = 0?":bool)
                            n259 = Equal To 0?(x=w287) -> (x = 0?=w290:bool)
                            n260 = Select(t=0.985 ("x"), s=w290, f=1.0) -> (s? t:f=w292:dbl)
                            n261 = Multiply(x=w292, y=w291) -> (x*y=w289:dbl)
                            n262 = Multiply(x=0.9, y=w287) -> (x*y=w288:dbl)
                            n263 = Add(x=w288, y=w289) -> (x+y=w307:dbl)
                            n264 = Multiply(x=w299, y=0.5) -> (x*y=w320:dbl)
                            n265 = In Range and Coerce(upper limit=w312, x=w307, lower limit=w311) -> (coerced(x)=w306:dbl)  [unwired: 1 out]
                            n266 = Add(x=w320, y=w321) -> (x+y=w293:dbl)
                            n267 = feedback-in #5(w306) -> ()
                            n268 = Absolute Value(x=w293) -> (abs(x)=w298:dbl)
                            n269 = Less?(x=w298, y=1e-06) -> (x < y?=w296:bool)
                            n270 = Select(t=0.0, s=w296, f=w293) -> (s? t:f=w294:dbl)
                            n271 = global write "G_VEH.vi" "handle"(w294) -> ()
                          }
                          frame Disabled {
                            n272 = flat-sequence {
                              tunnel: [w364] -> w333
                              frame #0 {
                                n273 = global read "G_VEH.vi" "candata"() -> (w363:T8)
                                n274 = Unbundle By Name(w363) -> ("VS_can"=w362:dbl)
                                n275 = Multiply(x=w362, y=0.5) -> (x*y=w360:dbl)
                                n276 = In Range and Coerce(upper limit=50.0, x=w360, lower limit=40.0) -> (coerced(x)=w357:dbl)  [unwired: 1 out]
                                n277 = Multiply(x=w357, y=w357) -> (x*y=w368:dbl)
                                n278 = Multiply(x=w357, y=w368) -> (x*y=w370:dbl)
                                n279 = Multiply(x=w368, y=0.5) -> (x*y=w365:dbl)
                                n280 = Divide(x=w370, y=3.0) -> (x/y=w366:dbl)
                                n281 = Build Array(w366, w365, w357) -> (w364:dbl[])
                              }
                            }
                            n282 = flat-sequence {
                              tunnel: [w348] -> w341
                              tunnel: [w343] -> w327
                              frame #0 {
                                n283 = global read "G_SEN.vi" "Lane_R_M"() -> (w351:dbl[])
                                n284 = global read "G_SEN.vi" "Lane_L_M"() -> (w352:dbl[])
                                n285 = Multiply(x=w352, y=0.5) -> (x*y=w355:dbl[])
                                n286 = Multiply(x=w351, y=0.5) -> (x*y=w356:dbl[])
                                n287 = Add(x=w355, y=w356) -> (x+y=w347:dbl[])
                                n288 = global write "G_SEN.vi" "Lane_C_I"(w347) -> ()
                                n289 = Index Array(array=w347, index=0) -> (element=w345:dbl)
                                n290 = Array Subset(array=w347, index=1, length=3) -> (w348:dbl[])
                                n291 = Less?(x=w345, y=0.8) -> (x < y?=w343:bool)
                              }
                            }
                            n292 = Multiply(x=w341, y=w333) -> (x*y=w342:dbl[])
                            n293 = Add Array Elements(numeric array=w342) -> (sum=w332:dbl)
                            n294 = global read "G_VEH.vi" "candata"() -> (w329:T8)
                            n295 = Select(t=0.0, s=w327, f=w332) -> (s? t:f=w331:dbl)
                            n296 = Unbundle By Name(w329) -> ("Steer_output"=w328:dbl)
                            n297 = Multiply(x=-0.2, y=w331) -> (x*y=w339:dbl)
                            n298 = Multiply(x=w339, y=0.1 ("x")) -> (x*y=w337:dbl)
                            n299 = Multiply(x=0.9, y=w328) -> (x*y=w336:dbl)
                            n300 = Add(x=w337, y=w336) -> (x+y=w335:dbl)
                            n301 = global write "G_VEH.vi" "handle"(w335) -> ()
                          }
                        }
                      }
                      frame #2 {
                        n302 = global read "G_VEH.vi" "candata"() -> (w379:T8)
                        n303 = Unbundle By Name(w379) -> ("VS_can"=w378:dbl)
                        n304 = Multiply(x=w378, y=0.9) -> (x*y=w376:dbl)
                        n305 = Max & Min(x=10.0, y=w376) -> (max(x,y)=w373:dbl)  [unwired: 1 out]
                        n306 = Max & Min(x=w373, y="Max. Vel.") -> (min(x,y)=w371:dbl)  [unwired: 1 out]
                        n307 = Select(t=w371, s=w380, f="Max. Vel.") -> (s? t:f=w374:dbl)
                        n308 = call "collision_fixed_steer.vi"("obsclose"="obs", "Max. Vel."=w374) -> ("collision"=w382:bool, "speed limit"=→"Speed limit":dbl)  [unwired: 8 in]
                        "collision" <- w382
                        n309 = Boolean To (0,1)(Boolean=w382) -> (0, 1=→"col":i16)
                      }
                      frame #3 {
                        n310 = global read "G_PATH.vi" "Mission"() -> (w385:i32)
                        "Mission" <- w385
                        n311 = case shown="9" w385 {
                          frame 0, Default {
                          }
                          frame 9 {
                            n312 = flat-sequence {
                              frame #0 {
                                n313 = global write "G_PATH.vi" "parking_cost"(0 ("parkingcost")) -> ()
                                n314 = global write "G_VEH.vi" "xparking"(T9 {"c_idx"=-1, "xc"=0.0, "yc"=0.0, "hc"=0.0, "xc_path"=0.0} ("xparking")) -> ()
                                n315 = global write "G_PATH.vi" "wpt_park"(dbl[][] [] ("wpt_park")) -> ()
                              }
                              frame #1 {
                                n316 = global read "G_PATH.vi" "path_rev"() -> (w389:dbl[][])
                                n317 = Empty Array?(array=w389) -> (empty?=w390:bool)
                                n318 = case shown="False" w390 {
                                frame False {
                                n319 = flat-sequence {
                                frame #0 {
                                n320 = disable-structure shown="Enabled" {
                                frame Enabled {
                                n321 = global read "G_PATH.vi" "path_rev"() -> (w396:dbl[][])
                                n322 = global read "G_VEH.vi" "xyhp"() -> (w391:T5)
                                n323 = Empty Array?(array=w396) -> (empty?=w395:bool)
                                n324 = Unbundle By Name(w391) -> ("idx"=w397:i32)
                                n325 = Not(x=w395) -> (.not. x?=w394:bool)
                                n326 = Equal To 0?(x=w397) -> (x = 0?=w393:bool)
                                n327 = And(x=w394, y=w393) -> (x .and. y?=w392:bool)
                                n328 = case shown="True" w392 {
                                frame False {
                                }
                                frame True {
                                n329 = flat-sequence {
                                tunnel: [w401] -> w398
                                frame #0 {
                                n330 = global read "G_PATH.vi" "path_rev"() -> (w399:dbl[][])
                                n331 = global write "G_PATH.vi" "path"(w399) -> ()
                                n332 = global write "G_PATH.vi" "path_origin"(w399) -> ()
                                }
                                frame #1 {
                                n333 = call "whereami.vi"() -> ()  [unwired: 12 in]
                                }
                                frame #2 {
                                n334 = global read "G_PATH.vi" "path"() -> (w400:dbl[][])
                                n335 = global read "G_VEH.vi" "xyhc"() -> (w402:T5)
                                n336 = call "findcurrentpointinpath.vi"("xyhc_in"=w402, "path_updated"=w400) -> ("xyhc_out"=w401:T5)  [unwired: 8 in, 1 out]
                                }
                                }
                                n337 = global write "G_VEH.vi" "xyhc"(w398) -> ()
                                }
                                }
                                }
                                frame Disabled {
                                }
                                }
                                }
                                frame #1 {
                                n338 = global read "G_VEH.vi" "xparking"() -> (w423:T5)
                                n339 = global read "G_NAV.vi" "M6006"() -> (w422:T7)
                                n340 = Unbundle By Name(w422) -> ("lcc[1]"=w420:dbl, "lcc[0]"=w418:dbl)
                                n341 = Unbundle By Name(w423) -> ("x"=w421:dbl, "y"=w419:dbl)
                                n342 = Subtract(x=w421, y=w420) -> (x-y=w417:dbl)
                                n343 = Subtract(x=w419, y=w418) -> (x-y=w416:dbl)
                                n344 = global read "G_VEH.vi" "candata"() -> (w410:T8)
                                n345 = Square(x=w417) -> (x^2=w415:dbl)
                                n346 = Square(x=w416) -> (x^2=w414:dbl)
                                n347 = Unbundle By Name(w410) -> ("VS_can"=w409:dbl)
                                n348 = Add(x=w415, y=w414) -> (x+y=w413:dbl)
                                n349 = Absolute Value(x=w409) -> (abs(x)=w408:dbl)
                                n350 = Square Root(x=w413) -> (sqrt(x)=w412:dbl)
                                n351 = global read "G_VEH.vi" "firstcall"() -> (w403:bool)
                                n352 = Less?(x=w412, y=1.2) -> (x < y?=w406:bool)
                                n353 = Less?(x=w408, y=0.05) -> (x < y?=w405:bool)
                                n354 = Compound Arithmetic op=AND(w403, w406, w405) -> (w404:bool)
                                n355 = case shown="False" w404 {
                                tunnel: w412 -> [w424 _]
                                frame False {
                                n356 = global read "G_SEN.vi" "sensor_etc"() -> (w427:dbl[][])
                                n357 = global read "G_VEH.vi" "candata"() -> (w434:T8)
                                n358 = Unbundle By Name(w434) -> ("VS_can"=w433:dbl)
                                n359 = Empty Array?(array=w427) -> (empty?=w426:bool)
                                n360 = In Range and Coerce(upper limit=6.0, x=w424, lower limit=1.5) -> (In Range?=w432:bool)  [unwired: 1 out]
                                n361 = Less Or Equal To 0?(x=w433) -> (x <= 0?=w431:bool)
                                n362 = Not(x=w426) -> (.not. x?=w425:bool)
                                n363 = Compound Arithmetic op=AND(w431, w432, w425) -> (w430:bool)
                                n364 = case shown="True" w430 {
                                frame False {
                                }
                                frame True {
                                n365 = global write "G_VEH.vi" "firstcall"(TRUE ("firstcall")) -> ()
                                n366 = call "parking_ung2rev.vi"() -> ()  [unwired: 12 in]
                                }
                                }
                                }
                                frame True {
                                n367 = flat-sequence {
                                frame #0 {
                                n368 = global write "G_VEH.vi" "parking_loop"(TRUE ("parking_loop")) -> ()
                                n369 = global write "G_VEH.vi" "firstcall"(FALSE ("firstcall")) -> ()
                                }
                                frame #1 {
                                n370 = call "parking_ung2_loop.vi"() -> ()  [unwired: 12 in]
                                }
                                }
                                }
                                }
                                }
                                }
                                }
                                frame True {
                                n371 = global read "G_VEH.vi" "xmission"() -> (w451:T5)
                                n372 = global read "G_NAV.vi" "M6006"() -> (w450:T7)
                                n373 = global write "G_VEH.vi" "parking_loop"(FALSE ("parking_loop")) -> ()
                                n374 = global write "G_VEH.vi" "firstcall"(TRUE ("firstcall")) -> ()
                                n375 = Unbundle By Name(w450) -> ("lcc[1]"=w448:dbl, "lcc[0]"=w446:dbl)
                                n376 = Unbundle By Name(w451) -> ("x"=w449:dbl, "y"=w447:dbl)
                                n377 = Subtract(x=w449, y=w448) -> (x-y=w445:dbl)
                                n378 = Subtract(x=w447, y=w446) -> (x-y=w444:dbl)
                                n379 = Square(x=w445) -> (x^2=w443:dbl)
                                n380 = Square(x=w444) -> (x^2=w442:dbl)
                                n381 = Add(x=w443, y=w442) -> (x+y=w441:dbl)
                                n382 = Square Root(x=w441) -> (sqrt(x)=w440:dbl)
                                n383 = Greater?(x=w440, y=5.0) -> (0:w438:bool)
                                n384 = case shown="True" w438 {
                                frame False {
                                }
                                frame True {
                                n385 = call "parking_ung2.vi"() -> ()  [unwired: 12 in]
                                }
                                }
                                }
                                }
                              }
                            }
                          }
                        }
                      }
                    }
                  }
                  frame True {
                    n386 = flat-sequence {
                      frame #0 {
                        w455 = FALSE ("X Scale.Loose Fit")
                        w454 = u8 0 ("X Scale.Scale Fit")
                        n387 = call "initvar.vi"() -> ()  [unwired: 12 in]
                        n388 = property on="XY Graph" class="XYGraph (strict)"("XScale.ScaleFit"=w454, "YScale.ScaleFit"=w454, "XScale.LooseFit"=w455, "YScale.LooseFit"=w455) -> ()  [unwired: 2 in, 2 out]
                      }
                      frame #1 {
                        n389 = global read "G_VEH.vi" "Location"() -> (w456:i32)
                        n390 = Bundle("Minimum"=-22.6, "Minimum"=22.6, "Minimum"=10.0, "Minimum"=1.0, "Minimum"=-20.0) -> (w469:T11)  [unwired: 1 in]
                        n391 = Bundle("Minimum"=-5.0, "Minimum"=37.3, "Minimum"=10.0, "Minimum"=1.0, "Minimum"=-20.0) -> (w462:T11)  [unwired: 1 in]
                        n392 = property on="XY Graph" class="XYGraph (strict)"("XScale.Range"=w469) -> ()  [unwired: 2 in, 2 out]
                        n393 = property on="XY Graph" class="XYGraph (strict)"("YScale.Range"=w462) -> ()  [unwired: 2 in, 2 out]
                        n394 = call "getecefdcmref.vi"("map"=w456) -> ("XYZ"=w457:dbl[])  [unwired: 10 in, 4 out]
                        n395 = global write "G_NAV.vi" "ecef ref"(w457) -> ()
                      }
                      frame #2 {
                        n396 = global read "G_DATA.vi" "path"() -> (w473:path)
                        n397 = Build Path(base path=w473, name or relative path="wpt") -> (appended path=w471:path)
                        n398 = call "Read From Measurement File2"("Filename"=w471, "Reset"=TRUE) -> ("error out"=w475:errorcluster, "Filename Out"=w470:path, "Signals"=w477:dynamicdata)  [unwired: 4 in, 3 out]
                        n399 = Unbundle By Name(w475) -> ("status"=w474:bool)
                        n400 = case shown="False" w474 {
                          tunnel: w477 -> [w479 _]
                          tunnel: w470 -> [w478 _]
                          frame False {
                            n401 = call "Convert from Dynamic Data2"("Dynamic Data Type"=w479) -> ("Array"=w481:dbl[][])  [unwired: 3 in]
                            n402 = Empty Array?(array=w481) -> (empty?=w480:bool)
                            n403 = case shown="False" w480 {
                              tunnel: w481 -> [w483 _]
                              tunnel: w478 -> [w482 _]
                              frame False {
                                n404 = call "path_ini_new.vi"("Filename Out"=w482, "WPT"=w483) -> ()  [unwired: 10 in]
                              }
                              frame True {
                                w484 = T12 [] ("Missions_origin")
                                w485 = dbl[][] [] ("path_updated")
                                n405 = global write "G_PATH.vi" "path"(w485) -> ()
                                n406 = global write "G_PATH.vi" "path_very_origin"(w485) -> ()
                                n407 = global write "G_PATH.vi" "path_origin"(w485) -> ()
                                n408 = global write "G_PATH.vi" "Missions_origin"(w484) -> ()
                                n409 = global write "G_PATH.vi" "Missions"(w484) -> ()
                              }
                            }
                          }
                          frame True {
                          }
                        }
                      }
                      frame #3 {
                        n410 = disable-structure shown="Disabled" {
                          disable-tunnel: [w487 _] -> w486
                          frame Disabled {
                            n411 = disable-structure shown="Enabled" {
                              disable-tunnel: [w493 _] -> w490
                              disable-tunnel: [w491 errorcluster {"status"=TRUE, "code"=0, "source"=""} ("error out")] -> w489
                              frame Enabled {
                                n412 = call "Read From Measurement File"("Reset"=TRUE) -> ("error out"=w491:errorcluster, "Signals"=w493:dynamicdata)  [unwired: 5 in, 4 out]
                              }
                              frame Disabled {
                              }
                            }
                            n413 = Unbundle By Name(w489) -> ("status"=w488:bool)
                            n414 = case shown="False" w488 {
                              tunnel: w490 -> [w499 _]
                              tunnel: [w495 _] -> w487
                              frame False {
                                n415 = call "Convert from Dynamic Data"("Dynamic Data Type"=w499) -> ("Array"=w496:dbl[][])  [unwired: 3 in]
                                n416 = for {
                                tunnel: w496 -> [w507] mode=indexing
                                tunnel: [w501] -> w497 mode=indexing
                                w500 = T5 {"idx"=0, "x"=0.0, "y"=0.0, "h"=0.0, "x_path"=0.0}  # x
                                n417 = Index Array(array=w507, index #1=0 ("index")) -> (element #1=w505:dbl, element #2=w504:dbl, element #3=w503:dbl)  [unwired: 2 in]
                                n418 = Bundle By Name(cluster=w500, "idx"=w505, "x"=w504, "y"=w503) -> (w502:T5)
                                n419 = Build Cluster Array(w502) -> (w501:T13)
                                }
                                n420 = Index Array(array=w497, index (col)=0 ("disabled index (col)")) -> (element=w495:T13)  [unwired: 1 in]
                              }
                              frame True {
                              }
                            }
                          }
                          frame Enabled {
                          }
                        }
                        n421 = global write "G_PATH.vi" "Missions_origin"(w486) -> ()
                        n422 = global write "G_PATH.vi" "Missions"(w486) -> ()
                      }
                      frame #4 {
                        n423 = global read "G_VEH.vi" "Location"() -> (w508:i32)
                        n424 = local write "Load WPT"(FALSE ("Load WPT")) -> ()
                        n425 = call "mapconf.vi"("Location"=w508) -> ("y"=w510:cluster{dbl, dbl, "y":dbl, "y":dbl, dbl}, "x"=w511:cluster{dbl, dbl, "y":dbl, "y":dbl, dbl}, "new picture"=w512:picture)  [unwired: 8 in]
                        n426 = property on="XY Graph 2" class="XYGraph (strict)"("PlotImages.Back"=w512) -> ()  [unwired: 2 in, 2 out]
                        n427 = property on="XY Graph 2" class="XYGraph (strict)"("XScale.Range"=w511, "YScale.Range"=w510) -> ()  [unwired: 2 in, 2 out]
                      }
                    }
                  }
                }
              }
              frame True {
                n428 = flat-sequence {
                  tunnel: [w519] -> w513
                  tunnel: w513 -> [w608]
                  frame #0 {
                    w514 = 0.0
                    n429 = disable-structure shown="Enabled" {
                      frame Disabled {
                        w515 = TRUE ("X Scale.Loose Fit")
                        w516 = u8 2 ("X Scale.Scale Fit")
                        n430 = property on="XY Graph" class="XYGraph (strict)"("XScale.ScaleFit"=w516, "YScale.ScaleFit"=w516, "XScale.LooseFit"=w515, "YScale.LooseFit"=w515) -> ()  [unwired: 2 in, 2 out]
                      }
                      frame Enabled {
                      }
                    }
                    n431 = global write "G_VEH.vi" "handle"(w514) -> ()
                    n432 = global write "G_VEH.vi" "VS_des"(w514) -> ()
                  }
                  frame #1 {
                    n433 = local read "Make WPT"() -> (w518:bool)
                    n434 = global read "G_VEH.vi" "Location"() -> (w517:i32)
                    n435 = Initialize Array(0.0 ("element"), 7 ("dimension size"), 1 ("dimension size")) -> (w520:dbl[][])
                    n436 = while {
                      shift-right: [w525] -> w519
                      shift-left: w520 -> [w527]
                      shift-right: [FALSE] -> _
                      shift-left: w518 -> [w528]
                      tunnel: w517 -> [w524]
                      stop <- w530 stop-if-true
                      n437 = flat-sequence {
                        tunnel: [w540] -> w526
                        tunnel: w524 -> [w533]
                        frame #0 {
                          n438 = global read "G_NAV.vi" "GPS_status"() -> (w532:T14)
                          n439 = disable-structure shown="Enabled" {
                            disable-tunnel: [w551 w555] -> w543
                            disable-tunnel: [w550 w554] -> w542
                            disable-tunnel: [w544 w553] -> w541
                            disable-tunnel: w532 -> [w549 w563]
                            disable-tunnel: [w548 w562] -> w539
                            disable-tunnel: [w547 w561] -> w538
                            disable-tunnel: [w544 w560] -> w537
                            disable-tunnel: w533 -> [_ w559]
                            frame Enabled {
                              n440 = global read "G_NAV.vi" "M6006"() -> (w552:T7)
                              n441 = Unbundle By Name(w552) -> ("lcc[0]"=w546:dbl, "lcc[1]"=w545:dbl)
                              n442 = Unbundle By Name(w549) -> ("lat"=w548:dbl, "lon"=w547:dbl, "hgt"=w544:dbl)
                              n443 = To Double Precision Float(number=w546) -> (double precision float=w551:dbl)
                              n444 = To Double Precision Float(number=w545) -> (double precision float=w550:dbl)
                            }
                            frame Disabled {
                              n445 = Unbundle By Name(w563) -> ("lat"=w562:dbl, "lon"=w561:dbl, "hgt"=w560:dbl)
                              n446 = call "getecefdcmref.vi"("map"=w559) -> ("XYZ"=w558:dbl[])  [unwired: 10 in, 4 out]
                              n447 = call "llh2lcc.vi"("ecef ref"=w558, "hgt"=w560, "lon"=w561, "lat"=w562) -> ("lcc"=w557:dbl[])  [unwired: 7 in]
                              n448 = Index Array(array=w557, index #1=0 ("index")) -> (element #1=w555:dbl, element #2=w554:dbl, element #3=w553:dbl)  [unwired: 2 in]
                            }
                          }
                          n449 = global read "G_VEH.vi" "candata"() -> (w536:T8)
                          n450 = Unbundle By Name(w536) -> ("VS_can"=w535:dbl)
                          n451 = To Double Precision Float(number=w533) -> (double precision float=w534:dbl)
                          n452 = Build Array(w539, w538, w537, w543, w542, w541, w535, w534) -> (w540:dbl[])
                        }
                      }
                      n453 = local read "Make WPT"() -> (w531:bool)
                      n454 = Not(x=w531) -> (.not. x?=w530:bool)
                      n455 = case shown="False" w528 {
                        tunnel: w527 -> [w578 w595]
                        tunnel: w526 -> [w577 w593]
                        tunnel: [w576 w592] -> w525
                        frame False {
                          n456 = Array Size(array=w578) -> (size(s)=w586:i32[])
                          n457 = Index Array(array=w586, index=1) -> (element=w575:i32)
                          n458 = Decrement(x=w575) -> (x-1=w574:i32)
                          n459 = Index Array(array=w578, index (col)=w574) -> (element=w582:dbl[])  [unwired: 1 in]
                          n460 = Index Array(array=w582, index #1=3 ("index"), index #2=4 ("index")) -> (element #1=w573:dbl, element #2=w571:dbl)
                          n461 = Index Array(array=w577, index #1=3 ("index"), index #2=4 ("index")) -> (element #1=w572:dbl, element #2=w570:dbl)
                          n462 = Subtract(x=w573, y=w572) -> (x-y=w569:dbl)
                          n463 = Subtract(x=w571, y=w570) -> (x-y=w568:dbl)
                          n464 = Square(x=w569) -> (x^2=w567:dbl)
                          n465 = Square(x=w568) -> (x^2=w566:dbl)
                          n466 = Add(x=w567, y=w566) -> (x+y=w565:dbl)
                          n467 = Greater Or Equal?(x=w565, y=0.25) -> (x >= y?=w579:bool)
                          n468 = case shown="True" w579 {
                            tunnel: w578 -> [w587 w591]
                            tunnel: w575 -> [_ w588]
                            tunnel: w577 -> [_ w590]
                            tunnel: [w587 w589] -> w576
                            frame False {
                            }
                            frame True {
                              n469 = Insert Into Array(array=w591, index (col)=w588, new element=w590) -> (w589:dbl[][])  [unwired: 1 in]
                            }
                          }
                        }
                        frame True {
                          n470 = Replace Array Subset(array=w595, new element=w593, index (col)=0 ("disabled index (col)")) -> (w592:dbl[][])  [unwired: 1 in]
                        }
                      }
                    }
                  }
                  frame #2 {
                    n471 = call "Convert to Dynamic Data"("2D Array"=w608) -> ("Dynamic Data Type"=w609:dynamicdata)  [unwired: 3 in]
                    n472 = global read "G_VEH.vi" "Location"() -> (w605:i32)
                    n473 = case shown="9" w605 {
                      tunnel: ["" ("String") "Hyundai" ("String") "KAIST" ("String") "AJOU" ("String") "MUNJI" ("String") "Airforce" ("String") "CAR" ("String") "KATRI" ("String") _ "coex" ("String")] -> w604
                      frame 0, Default {
                      }
                      frame 1 {
                      }
                      frame 2 {
                      }
                      frame 3 {
                      }
                      frame 4 {
                      }
                      frame 5 {
                      }
                      frame 6 {
                      }
                      frame 7 {
                      }
                      frame 8 {
                      }
                      frame 9 {
                      }
                    }
                    n474 = Get Date/Time In Seconds() -> (seconds since 1Jan1904=w606:timestamp)
                    n475 = Format Date/Time String(time format string (%c)="%2y%2m%2d%2H%2M", seconds (now)=w606) -> (date/time string=w602:string)  [unwired: 1 in]
                    n476 = global read "G_DATA.vi" "path"() -> (w600:path)
                    n477 = Build Path(base path=w600, name or relative path="wpt") -> (appended path=w598:path)
                    n478 = Concatenate Strings(w602, "_" ("string"), w604, ".lvm" ("string")) -> (w597:string)
                    n479 = Build Path(base path=w598, name or relative path=w597) -> (appended path=w596:path)
                    n480 = call "save wpt"("Signals"=w609, "Reset"=TRUE, "Filename"=w596) -> ()  [unwired: 14 in, 3 out]
                  }
                }
              }
            }
          }
        }
      }
    }
  }
  n481 = disable-structure shown="Enabled" {
    frame Enabled {
      n482 = flat-sequence {
        frame #0 {
          n483 = local write "obs"(FALSE ("obs")) -> ()
          n484 = local write "log"(TRUE ("obs")) -> ()
        }
        frame #1 {
          n485 = while {
            stop <- FALSE stop-if-true
            n486 = flat-sequence {
              frame #0 {
                n487 = Wait Until Next ms Multiple(millisecond multiple=u32 100 ("milliseconds to wait")) -> (millisecond timer value=w626:u32)
                n488 = feedback #7() -> (w624:u32)  [unwired: 1 in]
                n489 = feedback-in #7(w626) -> ()
                n490 = Subtract(x=w626, y=w624) -> (x-y=→"timmer":u32)
              }
              frame #1 {
                n491 = disable-structure shown="Enabled" {
                  frame Enabled {
                    n492 = case shown="False" "log" {
                      frame False {
                        n493 = global write "G_SEN.vi" "sensor_obs_log"(dbl[][] [] ("sensor_obs_log")) -> ()
                      }
                      frame True {
                        (unwired) 0.0 ("f")
                        n494 = call "obslog.vi"("xmax"=8.0, "xmin"=-5.0, "FF"=0.97 ("t"), "ymin"=0.0, "ymax"=20.0) -> ()  [unwired: 7 in]
                      }
                    }
                  }
                  frame Disabled {
                  }
                }
              }
              frame #2 {
                n495 = disable-structure shown="Enabled" {
                  frame Disabled {
                  }
                  frame Enabled {
                    n496 = disable-structure shown="Enabled" {
                      frame Disabled {
                        n497 = global read "G_PATH.vi" "RXY"() -> (w651:dbl[])
                        n498 = Index Array(array=w651) -> (element=w650:dbl)  [unwired: 1 in]
                        n499 = feedback #8(0.0 ("t")) -> (w642:dbl)
                        n500 = Greater?(x=w650, y=600.0) -> (0:w634:bool)
                        n501 = Multiply(x=0.95, y=w642) -> (x*y=w638:dbl)
                        n502 = Select(s=w634, f=i16 0) -> (s? t:f=w646:i16)  [unwired: 1 in]
                        n503 = Greater?(x=w638, y=0.01) -> (0:w639:bool)
                        n504 = Select(t=w638, s=w639, f=0.0) -> (s? t:f=w636:dbl)
                        n505 = Greater?(x=w646, y=i16 300) -> (0:w645:bool)
                        n506 = Select(t=1.0, s=w645, f=w636) -> (s? t:f=w635:dbl)
                        n507 = feedback-in #8(w635) -> ()
                        n508 = global write "G_SEN.vi" "crosswalk"(w635) -> ()
                      }
                      frame Enabled {
                        n509 = call "lanelog.vi"() -> ()  [unwired: 12 in]
                      }
                    }
                  }
                }
              }
              frame #3 {
                n510 = disable-structure shown="Enabled" {
                  frame Enabled {
                    n511 = disable-structure shown="Enabled" {
                      disable-tunnel: [w653 TRUE] -> w652
                      frame Disabled {
                        n512 = global read "G_PATH.vi" "xxx"() -> (w654:dbl)
                        n513 = Equal To 0?(x=w654) -> (x = 0?=w653:bool)
                      }
                      frame Enabled {
                      }
                    }
                    n514 = case shown="True" w652 {
                      frame False {
                      }
                      frame True {
                        n515 = call "newlane2.vi"("predict"=TRUE) -> ()  [unwired: 11 in]
                      }
                    }
                  }
                  frame Disabled {
                  }
                }
              }
            }
          }
        }
      }
    }
    frame Disabled {
      n516 = flat-sequence {
        frame #0 {
          n517 = global write "G_VEH.vi" "pos_slam"(T15 [[1.0, 0.0, 0.0, 0.0], [0.0, 1.0, 0.0, 0.0], [0.0, 0.0, 1.0, 0.0], [0.0, 0.0, 0.0, 1.0]] ("pos_slam")) -> ()
          n518 = global write "G_SEN.vi" "keydata"(dbl[][] [] ("keydata")) -> ()
        }
        frame #1 {
          n519 = while {
            stop <- FALSE stop-if-true
            n520 = flat-sequence {
              frame #0 {
                n521 = Wait Until Next ms Multiple(millisecond multiple=u32 10) -> ()  [unwired: 1 out]
              }
              frame #1 {
                n522 = global read "G_VEH.vi" "xsensor"() -> (w672:T5)
                n523 = feedback-in #9(w672) -> ()
                n524 = feedback #9(T5 {"idx"=0, "x"=0.0, "y"=0.0, "h"=0.0, "x_path"=0.0} ("xsensor")) -> (w673:T5)
                n525 = global read "G_VEH.vi" "candata"() -> (w669:T8)
                n526 = global read "G_LCM.vi" "POS_T"() -> (w663:T10)
                n527 = Not Equal?(x=w672, y=w673) -> (x != y?=w671:T16)
                n528 = Unbundle By Name(w669) -> ("VS_can"=w668:dbl)
                n529 = Unbundle By Name(w663) -> ("dt"=w662:dbl)
                n530 = Cluster To Array(cluster=w671) -> (array=w670:bool[])
                n531 = Or Array Elements(Boolean array=w670) -> (logical OR=w666:bool)
                n532 = Greater Than 0?(x=w662) -> (x > 0?=w661:bool)
                n533 = Greater?(x=w668, y=5.0) -> (0:w665:bool)
                n534 = Compound Arithmetic op=AND(w666, w665, w661) -> (w664:bool)
                n535 = case shown="True" w664 {
                  frame False {
                  }
                  frame True {
                    n536 = flat-sequence {
                      frame #0 {
                      }
                      frame #1 {
                        n537 = global read "G_SEN.vi" "sensor_lane"() -> (w685:dbl[][])
                        n538 = global read "G_SEN.vi" "sensor_lane"() -> (w686:dbl[][])
                        n539 = global read "G_SEN.vi" "lane_log_R"() -> (w700:dbl[][])
                        n540 = global read "G_SEN.vi" "lane_log_L"() -> (w697:dbl[][])
                        n541 = global read "G_SEN.vi" "Lane_L_M"() -> (w679:dbl[])
                        n542 = global read "G_SEN.vi" "Lane_R_M"() -> (w680:dbl[])
                        n543 = global read "G_VEH.vi" "xsensor"() -> (w682:T5)
                        n544 = global read "G_VEH.vi" "xsensor"() -> (w681:T5)
                        n545 = call "lanelog2.vi"("xsensor"=w682, "thresh"=0.02, "lane_log"=w697, "sensor"=w685, "Lane_M"=w679) -> ("lane_log_out"=w698:dbl[][], "sensor_out"=w676:dbl[][], "lane_I_out"=w683:dbl[])  [unwired: 2 in, 2 out]
                        n546 = call "lanelog2.vi"("xsensor"=w681, "thresh"=0.02, "lane_log"=w700, "sensor"=w686, "Lane_M"=w680) -> ("lane_log_out"=w699:dbl[][], "sensor_out"=w675:dbl[][], "lane_I_out"=w684:dbl[])  [unwired: 2 in, 2 out]
                        n547 = disable-structure shown="Disabled" {
                          disable-tunnel: w676 -> [w702 _]
                          frame Disabled {
                            n548 = call "Convert to Dynamic Data2"("2D Array"=w702) -> ("Dynamic Data Type"=w703:dynamicdata)  [unwired: 3 in]
                            n549 = call "Write To Measurement File"("Signals"=w703, "Filename"=path "left.lvm") -> ()  [unwired: 15 in, 3 out]
                          }
                          frame Enabled {
                          }
                        }
                        n550 = global write "G_SEN.vi" "lane_log_L"(w698) -> ()
                        n551 = disable-structure shown="Disabled" {
                          disable-tunnel: w675 -> [w704 _]
                          frame Disabled {
                            n552 = call "Convert to Dynamic Data3"("2D Array"=w704) -> ("Dynamic Data Type"=w705:dynamicdata)  [unwired: 3 in]
                            n553 = call "Write To Measurement File2"("Signals"=w705, "Filename"=path "right.lvm") -> ()  [unwired: 15 in, 3 out]
                          }
                          frame Enabled {
                          }
                        }
                        n554 = global write "G_SEN.vi" "lane_log_R"(w699) -> ()
                        n555 = Index Array(array=w683, index=0) -> (element=w694:dbl)
                        n556 = Index Array(array=w684, index=0) -> (element=w695:dbl)
                        n557 = Not Equal To 0?(x=w694) -> (x != 0?=w691:bool)
                        n558 = Not Equal To 0?(x=w695) -> (x != 0?=w692:bool)
                        n559 = Build Array(w692, w691) -> (w690:bool[])
                        n560 = Boolean Array To Number(Boolean array=w690) -> (number=w689:u32)
                        n561 = case shown="3" w689 {
                          tunnel: w684 -> [_ w747 _ w848]
                          tunnel: w683 -> [_ _ w789 w849]
                          tunnel: [w708 w746 w787 w840] -> w678
                          tunnel: [w707 w745 w788 w830] -> w677
                          frame 0, Default {
                            n562 = flat-sequence {
                              tunnel: [w709] -> w707
                              frame #0 {
                                w722 = 0.0 ("element")
                                n563 = global read "G_SEN.vi" "lane_width"() -> (w721:dbl)
                                n564 = global read "G_SEN.vi" "Lane_L_I"() -> (w715:dbl[])
                                n565 = Multiply(x=w721, y=-0.5) -> (x*y=w719:dbl)
                                n566 = Array Subset(array=w715, index=0, length=4) -> (w714:dbl[])
                                n567 = Build Array(w722, w722, w722, w719) -> (w718:dbl[])
                                n568 = global read "G_SEN.vi" "Lane_L_I"() -> (w713:dbl[])
                                n569 = Multiply(x=w714, y=0.975) -> (x*y=w724:dbl[])
                                n570 = Multiply(x=w718, y=0.025) -> (x*y=w723:dbl[])
                                n571 = Add(x=w724, y=w723) -> (x+y=w711:dbl[])
                                n572 = Array Subset(array=w713, index=4) -> (w710:dbl[])  [unwired: 1 in]
                                n573 = Build Array (concatenate)(w711, w710) -> (w709:dbl[])
                              }
                            }
                            n574 = flat-sequence {
                              tunnel: [w727] -> w708
                              frame #0 {
                                w740 = 0.0 ("element")
                                n575 = global read "G_SEN.vi" "lane_width"() -> (w741:dbl)
                                n576 = global read "G_SEN.vi" "Lane_R_I"() -> (w733:dbl[])
                                n577 = Multiply(x=w741, y=0.5) -> (x*y=w743:dbl)
                                n578 = Array Subset(array=w733, index=0, length=4) -> (w732:dbl[])
                                n579 = Build Array(w740, w740, w740, w743) -> (w744:dbl[])
                                n580 = global read "G_SEN.vi" "Lane_R_I"() -> (w731:dbl[])
                                n581 = Multiply(x=w732, y=0.975) -> (x*y=w738:dbl[])
                                n582 = Multiply(x=w744, y=0.025) -> (x*y=w739:dbl[])
                                n583 = Add(x=w738, y=w739) -> (x+y=w729:dbl[])
                                n584 = Array Subset(array=w731, index=4) -> (w728:dbl[])  [unwired: 1 in]
                                n585 = Build Array (concatenate)(w729, w728) -> (w727:dbl[])
                              }
                            }
                          }
                          frame 1 {
                            n586 = flat-sequence {
                              tunnel: w747 -> [w782]
                              tunnel: [w770] -> w746
                              frame #0 {
                                n587 = global read "G_SEN.vi" "Lane_R_I"() -> (w779:dbl[])
                                n588 = global read "G_VEH.vi" "xsensor"() -> (w777:T5)
                                n589 = To Double Precision Float(number=w777) -> (double precision float=w776:T17)
                                n590 = Array Subset(array=w779, index=0, length=4) -> (w778:dbl[])
                                n591 = Cluster To Array(cluster=w776) -> (array=w775:dbl[])
                                n592 = Multiply(x=w778, y=0.6) -> (x*y=w784:dbl[])
                                n593 = Multiply(x=w782, y=0.4) -> (x*y=w783:dbl[])
                                n594 = Add(x=w784, y=w783) -> (x+y=w771:dbl[])
                                n595 = Array Subset(array=w775, index=1, length=3) -> (w772:dbl[])
                                n596 = Build Array (concatenate)(w771, w772) -> (w770:dbl[])
                              }
                            }
                            n597 = flat-sequence {
                              tunnel: w747 -> [w762]
                              tunnel: [w748] -> w745
                              frame #0 {
                                n598 = global read "G_SEN.vi" "lane_width"() -> (w767:dbl)
                                n599 = Index Array(array=w762, index=3) -> (element=w768:dbl)
                                n600 = Subtract(x=w768, y=w767) -> (x-y=w765:dbl)
                                n601 = global read "G_SEN.vi" "Lane_L_I"() -> (w752:dbl[])
                                n602 = Replace Array Subset(array=w762, new element #1=w765, index #1=3 ("index"), new element #2=0.25 ("new element/subarray"), index #2=0 ("index")) -> (w757:dbl[])
                                n603 = Array Subset(array=w752, index=0, length=4) -> (w754:dbl[])
                                n604 = global read "G_SEN.vi" "Lane_L_I"() -> (w749:dbl[])
                                n605 = Multiply(x=w754, y=0.6) -> (x*y=w760:dbl[])
                                n606 = Multiply(x=w757, y=0.4) -> (x*y=w761:dbl[])
                                n607 = Add(x=w760, y=w761) -> (x+y=w751:dbl[])
                                n608 = Array Subset(array=w749, index=4) -> (w750:dbl[])  [unwired: 1 in]
                                n609 = Build Array (concatenate)(w751, w750) -> (w748:dbl[])
                              }
                            }
                          }
                          frame 2 {
                            n610 = flat-sequence {
                              tunnel: w789 -> [w804]
                              tunnel: [w790] -> w787
                              frame #0 {
                                n611 = global read "G_SEN.vi" "lane_width"() -> (w809:dbl)
                                n612 = Index Array(array=w804, index=3) -> (element=w810:dbl)
                                n613 = Add(x=w810, y=w809) -> (x+y=w807:dbl)
                                n614 = global read "G_SEN.vi" "Lane_R_I"() -> (w797:dbl[])
                                n615 = Replace Array Subset(array=w804, new element #1=w807, index #1=3 ("index"), new element #2=0.25 ("new element/subarray"), index #2=0 ("index")) -> (w799:dbl[])
                                n616 = Array Subset(array=w797, index=0, length=4) -> (w795:dbl[])
                                n617 = global read "G_SEN.vi" "Lane_R_I"() -> (w794:dbl[])
                                n618 = Multiply(x=w795, y=0.6) -> (x*y=w801:dbl[])
                                n619 = Multiply(x=w799, y=0.4) -> (x*y=w800:dbl[])
                                n620 = Add(x=w801, y=w800) -> (x+y=w791:dbl[])
                                n621 = Array Subset(array=w794, index=4) -> (w792:dbl[])  [unwired: 1 in]
                                n622 = Build Array (concatenate)(w791, w792) -> (w790:dbl[])
                              }
                            }
                            n623 = flat-sequence {
                              tunnel: w789 -> [w824]
                              tunnel: [w812] -> w788
                              frame #0 {
                                n624 = global read "G_SEN.vi" "Lane_L_I"() -> (w821:dbl[])
                                n625 = global read "G_VEH.vi" "xsensor"() -> (w819:T5)
                                n626 = To Double Precision Float(number=w819) -> (double precision float=w818:T17)
                                n627 = Array Subset(array=w821, index=0, length=4) -> (w820:dbl[])
                                n628 = Cluster To Array(cluster=w818) -> (array=w817:dbl[])
                                n629 = Multiply(x=w820, y=0.6) -> (x*y=w826:dbl[])
                                n630 = Multiply(x=w824, y=0.4) -> (x*y=w825:dbl[])
                                n631 = Add(x=w826, y=w825) -> (x+y=w814:dbl[])
                                n632 = Array Subset(array=w817, index=1, length=3) -> (w813:dbl[])
                                n633 = Build Array (concatenate)(w814, w813) -> (w812:dbl[])
                              }
                            }
                          }
                          frame 3 {
                            n634 = Subtract(x=w848, y=w849) -> (x-y=w851:dbl[])
                            n635 = Index Array(array=w851, index=3) -> (element=w846:dbl)
                            n636 = Greater?(x=w846, y=2.0) -> (0:w845:bool)
                            n637 = case shown="False" w845 {
                              tunnel: w849 -> [w861 w887]
                              tunnel: [w860 w879] -> w831
                              tunnel: w848 -> [w854 w881]
                              tunnel: [w853 w877] -> w841
                              tunnel: w846 -> [w852 _]
                              frame True {
                                n638 = global write "G_SEN.vi" "lane_width"(w852) -> ()
                                n639 = global read "G_SEN.vi" "Lane_R_I"() -> (w855:dbl[])
                                n640 = global read "G_SEN.vi" "Lane_L_I"() -> (w862:dbl[])
                                n641 = Multiply(x=w862, y=0.6) -> (x*y=w864:dbl[])
                                n642 = Multiply(x=w861, y=0.4) -> (x*y=w863:dbl[])
                                n643 = Multiply(x=w855, y=0.6) -> (x*y=w857:dbl[])
                                n644 = Multiply(x=w854, y=0.4) -> (x*y=w856:dbl[])
                                n645 = Add(x=w864, y=w863) -> (x+y=w860:dbl[])
                                n646 = Add(x=w857, y=w856) -> (x+y=w853:dbl[])
                              }
                              frame False {
                                n647 = global read "G_SEN.vi" "Lane_R_I"() -> (w882:dbl[])
                                n648 = global read "G_SEN.vi" "Lane_L_I"() -> (w888:dbl[])
                                n649 = Multiply(x=w888, y=0.6) -> (x*y=w890:dbl[])
                                n650 = Multiply(x=w887, y=0.4) -> (x*y=w889:dbl[])
                                n651 = Multiply(x=w882, y=0.6) -> (x*y=w884:dbl[])
                                n652 = Multiply(x=w881, y=0.4) -> (x*y=w883:dbl[])
                                n653 = Add(x=w890, y=w889) -> (x+y=w867:dbl[])
                                n654 = Add(x=w884, y=w883) -> (x+y=w876:dbl[])
                                n655 = Index Array(array=w867, index=0) -> (element=w870:dbl)
                                n656 = Index Array(array=w876, index=0) -> (element=w874:dbl)
                                n657 = Max & Min(x=w870, y=0.5 ("new element/subarray")) -> (min(x,y)=w868:dbl)  [unwired: 1 out]
                                n658 = Max & Min(x=w874, y=0.5 ("new element/subarray")) -> (min(x,y)=w872:dbl)  [unwired: 1 out]
                                n659 = Replace Array Subset(array=w867, new element=w868, index=0) -> (w879:dbl[])
                                n660 = Replace Array Subset(array=w876, new element=w872, index=0) -> (w877:dbl[])
                              }
                            }
                            n661 = global read "G_VEH.vi" "xsensor"() -> (w839:T5)
                            n662 = To Double Precision Float(number=w839) -> (double precision float=w838:T17)
                            n663 = Cluster To Array(cluster=w838) -> (array=w837:dbl[])
                            n664 = Array Subset(array=w841, index=0, length=4) -> (w842:dbl[])
                            n665 = Array Subset(array=w831, index=0, length=4) -> (w834:dbl[])
                            n666 = Array Subset(array=w837, index=1, length=3) -> (w829:dbl[])
                            n667 = Build Array (concatenate)(w842, w829) -> (w840:dbl[])
                            n668 = Build Array (concatenate)(w834, w829) -> (w830:dbl[])
                          }
                        }
                        n669 = global write "G_SEN.vi" "Lane_R_I"(w678) -> ()
                        n670 = global write "G_SEN.vi" "Lane_L_I"(w677) -> ()
                      }
                      frame #2 {
                        n671 = stacked-sequence {
                          frame #0 {
                            n672 = global read "G_SEN.vi" "Lane_R_I"() -> (w895:dbl[])
                            n673 = Array Subset(array=w895, index=0, length=4) -> (w894:dbl[])
                            n674 = while {
                              shift-right: [w967] -> _
                              shift-left: dbl[] [] ("lane_I_out") -> [w966]
                              shift-right: [w957] -> w908
                              shift-left: 0 ("size") -> [w964]
                              shift-right: [w962] -> w907
                              shift-left: w894 -> [w963]
                              stop <- w958 stop-if-true
                              n675 = Index Array(array=w963, index=3) -> (element=w975:dbl)
                              n676 = Add(x=w975, y=0.5) -> (x+y=w971:dbl)
                              n677 = global read "G_SEN.vi" "sensor_obs"() -> (w979:dbl[][])
                              n678 = global read "G_VEH.vi" "xsensor"() -> (w956:T5)
                              n679 = Replace Array Subset(array=w963, new element=w971, index=3) -> (w977:dbl[])
                              n680 = call "lanelog2.vi"("xsensor"=w956, "thresh"=0.025, "lane_log"=dbl[][] [], "sensor"=w979, "Lane_M"=w977) -> ("lane_I_out"=w968:dbl[], "lane_M_out"=w962:dbl[], "size"=w965:i32)  [unwired: 2 in, 2 out]
                              n681 = Greater?(x=w965, y=w964) -> (0:w969:bool)
                              n682 = Max & Min(x=w965, y=w964) -> (max(x,y)=w957:i32)  [unwired: 1 out]
                              n683 = Select(t=w968, s=w969, f=w966) -> (s? t:f=w967:dbl[])
                              n684 = Greater?(x=w971, y=8.0) -> (0:w959:bool)
                              n685 = Greater?(x=w957, y=50) -> (0:w960:bool)
                              n686 = Or(x=w959, y=w960) -> (x .or. y?=w958:bool)
                            }
                            n687 = flat-sequence {
                              tunnel: [w945] -> w906
                              tunnel: [w944] -> w905
                              tunnel: w894 -> [w942]
                              tunnel: [w941] -> w893
                              frame #0 {
                                n688 = global read "G_SEN.vi" "lane_width"() -> (w950:dbl)
                                n689 = Index Array(array=w942, index=3) -> (element=w951:dbl)
                                n690 = Add(x=w951, y=w950) -> (x+y=w948:dbl)
                                n691 = global read "G_SEN.vi" "lane_log_RR"() -> (w946:dbl[][])
                                n692 = global read "G_SEN.vi" "sensor_lane"() -> (w955:dbl[][])
                                n693 = global read "G_VEH.vi" "xsensor"() -> (w943:T5)
                                n694 = Replace Array Subset(array=w942, new element=w948, index=3) -> (w953:dbl[])
                                n695 = call "lanelog2.vi"("xsensor"=w943, "thresh"=0.025, "lane_log"=w946, "sensor"=w955, "Lane_M"=w953) -> ("lane_log_out"=w947:dbl[][], "sensor_out"=w941:dbl[][], "lane_I_out"=w945:dbl[], "size"=w944:i32)  [unwired: 2 in, 1 out]
                                n696 = global write "G_SEN.vi" "lane_log_RR"(w947) -> ()
                              }
                            }
                            n697 = disable-structure shown="Enabled" {
                              disable-tunnel: w908 -> [w924 w940]
                              disable-tunnel: [w922 w926] -> w899
                              disable-tunnel: w907 -> [w916 w933]
                              disable-tunnel: w906 -> [w915 w928]
                              disable-tunnel: w905 -> [_ w931]
                              frame Disabled {
                                n698 = Index Array(array=w916, index=3) -> (element=w919:dbl)
                                n699 = Index Array(array=w915, index=3) -> (element=w918:dbl)
                                n700 = Less?(x=w919, y=w918) -> (x < y?=w917:bool)
                                n701 = Select(t=w916, s=w917, f=w915) -> (s? t:f=w914:dbl[])
                                n702 = Greater?(x=w924, y=50) -> (0:w923:bool)
                                n703 = Select(t=w914, s=w923, f=w915) -> (s? t:f=w922:dbl[])
                              }
                              frame Enabled {
                                n704 = Greater?(x=w931, y=w940) -> (0:w939:bool)
                                n705 = Index Array(array=w928, index=3) -> (element=w936:dbl)
                                n706 = Index Array(array=w933, index=3) -> (element=w935:dbl)
                                n707 = Less?(x=w936, y=w935) -> (x < y?=w934:bool)
                                n708 = Select(t=w928, s=w934, f=w933) -> (s? t:f=w932:dbl[])
                                n709 = Select(t=w928, s=w939, f=w932) -> (s? t:f=w927:dbl[])
                                n710 = Greater?(x=w931, y=50) -> (0:w929:bool)
                                n711 = Select(t=w928, s=w929, f=w927) -> (s? t:f=w926:dbl[])
                              }
                            }
                            n712 = disable-structure shown="Disabled" {
                              disable-tunnel: w893 -> [w911 _]
                              frame Disabled {
                                n713 = call "Convert to Dynamic Data4"("2D Array"=w911) -> ("Dynamic Data Type"=w913:dynamicdata)  [unwired: 3 in]
                                n714 = call "Write To Measurement File3"("Signals"=w913, "Filename"=path "right2.lvm") -> ()  [unwired: 15 in, 3 out]
                              }
                              frame Enabled {
                              }
                            }
                            n715 = global read "G_SEN.vi" "Lane_RR_I"() -> (w900:dbl[])
                            n716 = Multiply(x=w900, y=0.8) -> (x*y=w902:dbl[])
                            n717 = Multiply(x=w899, y=0.2) -> (x*y=w901:dbl[])
                            n718 = Add(x=w902, y=w901) -> (x+y=w898:dbl[])
                            n719 = global write "G_SEN.vi" "Lane_RR_I"(w898) -> ()
                          }
                          frame #1 {
                            n720 = global read "G_SEN.vi" "Lane_L_I"() -> (w982:dbl[])
                            n721 = Array Subset(array=w982, index=0, length=4) -> (w981:dbl[])
                            n722 = while {
                              shift-right: [w1054] -> _
                              shift-left: dbl[] [] ("lane_I_out") -> [w1053]
                              shift-right: [w1044] -> w995
                              shift-left: 0 ("size") -> [w1051]
                              shift-right: [w1049] -> w994
                              shift-left: w981 -> [w1050]
                              stop <- w1045 stop-if-true
                              n723 = Index Array(array=w1050, index=3) -> (element=w1062:dbl)
                              n724 = Subtract(x=w1062, y=0.5) -> (x-y=w1058:dbl)
                              n725 = global read "G_SEN.vi" "sensor_obs"() -> (w1066:dbl[][])
                              n726 = global read "G_VEH.vi" "xsensor"() -> (w1043:T5)
                              n727 = Replace Array Subset(array=w1050, new element=w1058, index=3) -> (w1064:dbl[])
                              n728 = call "lanelog2.vi"("xsensor"=w1043, "thresh"=0.025, "lane_log"=dbl[][] [], "sensor"=w1066, "Lane_M"=w1064) -> ("lane_I_out"=w1055:dbl[], "lane_M_out"=w1049:dbl[], "size"=w1052:i32)  [unwired: 2 in, 2 out]
                              n729 = Greater?(x=w1052, y=w1051) -> (0:w1056:bool)
                              n730 = Max & Min(x=w1052, y=w1051) -> (max(x,y)=w1044:i32)  [unwired: 1 out]
                              n731 = Select(t=w1055, s=w1056, f=w1053) -> (s? t:f=w1054:dbl[])
                              n732 = Less?(x=w1058, y=-8.0) -> (x < y?=w1046:bool)
                              n733 = Greater?(x=w1044, y=50) -> (0:w1047:bool)
                              n734 = Or(x=w1046, y=w1047) -> (x .or. y?=w1045:bool)
                            }
                            n735 = flat-sequence {
                              tunnel: [w1032] -> w993
                              tunnel: [w1031] -> w992
                              tunnel: w981 -> [w1029]
                              tunnel: [w1028] -> w980
                              frame #0 {
                                n736 = global read "G_SEN.vi" "lane_width"() -> (w1037:dbl)
                                n737 = Index Array(array=w1029, index=3) -> (element=w1038:dbl)
                                n738 = Subtract(x=w1038, y=w1037) -> (x-y=w1035:dbl)
                                n739 = global read "G_SEN.vi" "lane_log_LL"() -> (w1033:dbl[][])
                                n740 = global read "G_SEN.vi" "sensor_lane"() -> (w1042:dbl[][])
                                n741 = global read "G_VEH.vi" "xsensor"() -> (w1030:T5)
                                n742 = Replace Array Subset(array=w1029, new element=w1035, index=3) -> (w1040:dbl[])
                                n743 = call "lanelog2.vi"("xsensor"=w1030, "thresh"=0.025, "lane_log"=w1033, "sensor"=w1042, "Lane_M"=w1040) -> ("lane_log_out"=w1034:dbl[][], "sensor_out"=w1028:dbl[][], "lane_I_out"=w1032:dbl[], "size"=w1031:i32)  [unwired: 2 in, 1 out]
                                n744 = global write "G_SEN.vi" "lane_log_LL"(w1034) -> ()
                              }
                            }
                            n745 = disable-structure shown="Enabled" {
                              disable-tunnel: w995 -> [w1011 w1027]
                              disable-tunnel: [w1009 w1013] -> w988
                              disable-tunnel: w994 -> [w1003 w1020]
                              disable-tunnel: w993 -> [w1002 w1015]
                              disable-tunnel: w992 -> [_ w1018]
                              frame Disabled {
                                n746 = Index Array(array=w1003, index=3) -> (element=w1006:dbl)
                                n747 = Index Array(array=w1002, index=3) -> (element=w1005:dbl)
                                n748 = Greater?(x=w1006, y=w1005) -> (0:w1004:bool)
                                n749 = Select(t=w1003, s=w1004, f=w1002) -> (s? t:f=w1001:dbl[])
                                n750 = Greater?(x=w1011, y=50) -> (0:w1010:bool)
                                n751 = Select(t=w1001, s=w1010, f=w1002) -> (s? t:f=w1009:dbl[])
                              }
                              frame Enabled {
                                n752 = Greater?(x=w1018, y=w1027) -> (0:w1026:bool)
                                n753 = Index Array(array=w1015, index=3) -> (element=w1023:dbl)
                                n754 = Index Array(array=w1020, index=3) -> (element=w1022:dbl)
                                n755 = Greater?(x=w1023, y=w1022) -> (0:w1021:bool)
                                n756 = Select(t=w1015, s=w1021, f=w1020) -> (s? t:f=w1019:dbl[])
                                n757 = Select(t=w1015, s=w1026, f=w1019) -> (s? t:f=w1014:dbl[])
                                n758 = Greater?(x=w1018, y=50) -> (0:w1016:bool)
                                n759 = Select(t=w1015, s=w1016, f=w1014) -> (s? t:f=w1013:dbl[])
                              }
                            }
                            n760 = disable-structure shown="Disabled" {
                              disable-tunnel: w980 -> [w998 _]
                              frame Disabled {
                                n761 = call "Convert to Dynamic Data5"("2D Array"=w998) -> ("Dynamic Data Type"=w999:dynamicdata)  [unwired: 3 in]
                                n762 = call "Write To Measurement File4"("Signals"=w999, "Filename"=path "left2.lvm") -> ()  [unwired: 15 in, 3 out]
                              }
                              frame Enabled {
                              }
                            }
                            n763 = global read "G_SEN.vi" "Lane_LL_I"() -> (w991:dbl[])
                            n764 = Multiply(x=w991, y=0.8) -> (x*y=w987:dbl[])
                            n765 = Multiply(x=w988, y=0.2) -> (x*y=w986:dbl[])
                            n766 = Add(x=w987, y=w986) -> (x+y=w985:dbl[])
                            n767 = global write "G_SEN.vi" "Lane_LL_I"(w985) -> ()
                          }
                        }
                      }
                    }
                  }
                }
              }
            }
          }
        }
      }
    }
  }
